vi "Query_Dust_Event.vi"(8 "error in (no error)":errorcluster, 9 "Save Waveforms":bool) -> (0 "error out":errorcluster)   [LabVIEW 2013]
uses:
  Private/Constraints.ctl
  Private/Graph.ctl
  <vilib>/Utility/miscctls.llb/LVPointTypeDef.ctl
  <vilib>/addons/database/Auxilliary.llb/DB Tools Cursor Type.ctl
  <vilib>/Utility/error.llb/DialogType.ctl
  <vilib>/addons/database/Connection.llb/Conn Execute.vi
  <vilib>/addons/database/Recordset.llb/Rec Fetch Recordset Data (R).vi
  <vilib>/addons/database/Recordset.llb/Rec Destroy - Connection.vi
  <userlib>/_OpenG.lib/array/array.llb/Remove Duplicates from 1D Array (String)__ogtk.vi
  <userlib>/_OpenG.lib/array/array.llb/Search 1D Array (String)__ogtk.vi
  <userlib>/_OpenG.lib/array/array.llb/Index 1D Array Elements (String)__ogtk.vi
  <userlib>/_OpenG.lib/array/array.llb/Filter 1D Array (String)__ogtk.vi
  <vilib>/Utility/file.llb/Write To Spreadsheet File (string).vi
  Private/Global graph.vi
  Private/throttle from query.vi
  <userlib>/_OpenG.lib/comparison/comparison.llb/1D String Array Changed__ogtk.vi
  <vilib>/addons/database/_DB Variant To Data/Database Variant To Data.xnode
  <vilib>/addons/database/NI_Database_API.lvlib
panel:
  out "Last Metadata Name":string
  out "Current Limits":T1 {"Dust Quality" scale=0.0..5.0}
  out "Density":dbl
  out "Plotted Cluster":T2 {"Estimate Quality" scale=0.0..5.0; "Lower Mass Limit (kg)" min=-1.0 max=1.0 step=1e-20; "Upper Mass Limit (kg)" min=-1.0 max=1.0 step=1e-20; "Lower Velocity Limit (km/s)" min=-1.0 max=299792000.0; "Upper Velocity Limit (km/s)" min=-1.0 max=299792000.0}
  out "Groups to add":string[](array[string])
  out "Experiments\nto add":string[](array[string])
  out "Reset":bool
  out "Run stop integer timesamp Holder":i64[](array[numeric])
  out "Run start integer timestamp Holder":i64[](array[numeric])
  out "Description Holder":string[](array[string])
  out "Names":string[](array[string])
  in  "write metadata only":bool
  in  "Tab Control":T3(tab)
  in  "Reset Scale to Default":bool
  in  "Reset Limit":bool
  in  "Combine":bool
  out "Plotted Experiment Names":i32(listbox)
  out "Plotted Experiment Groups":i32(listbox)
  in  "Clear Extra Plots":bool
  in  "Experiment Group":string
  in  "Plot":bool
  in  "Search":bool
  in  "Throttle Dust Source After:":i64=9223372036854775807
  in  "Select Names":bool
  in  "Save Metadata":bool
  in  "Show Names":bool
  out "metadata Slide":u8(slide) scale=0.0..100.0
  in  "Save Image":bool
  in  "Plot Radius?":bool
  out "Constrained Distribution":T4
  in  "Experiment Name":string
  out "Slide":u8(slide) scale=0.0..100.0
  in  "Update Plot in Real-time?":bool
  in  "Reset Constraints to Default":bool
  in  "New Plot Window":bool
  out "Number of Matching Events:":i32
  out "Description for Experiment Name:":string caption="Experiment Description:"
  out "Percentage of triggers that fit constraints:":dbl format="%#_4g%"
  out "Total Number of triggers:":i64
  in  "Constraints":T2 {"Estimate Quality" scale=0.0..5.0; "Lower Mass Limit (kg)" min=0.0 step=1e-20; "Upper Mass Limit (kg)" min=0.0 step=1e-20}
  out "Dust Type":string
  in  "Radius (µm)":dbl
  in  "Mass":dbl
  in  "Velocity":dbl
  in  "Update interval (s)":dbl=10.0 min=10.0 max=120.0
  in  "Sensitivity:":dbl=12100000000000.0
  in  "Vnoise Estimate:":dbl=0.005
  in  "Pelletron Voltage (MV):":dbl=2.0
  out "Test":bool caption="Test Database in use:"
  out "Test 2":bool caption="Production Database in use:"
  in  "Exit":bool
  # "Query Dust Event"
  # "Cursor"
  # "Plot Settings:"
  # "Error Status:"
  # "ODBC Connection Status:"
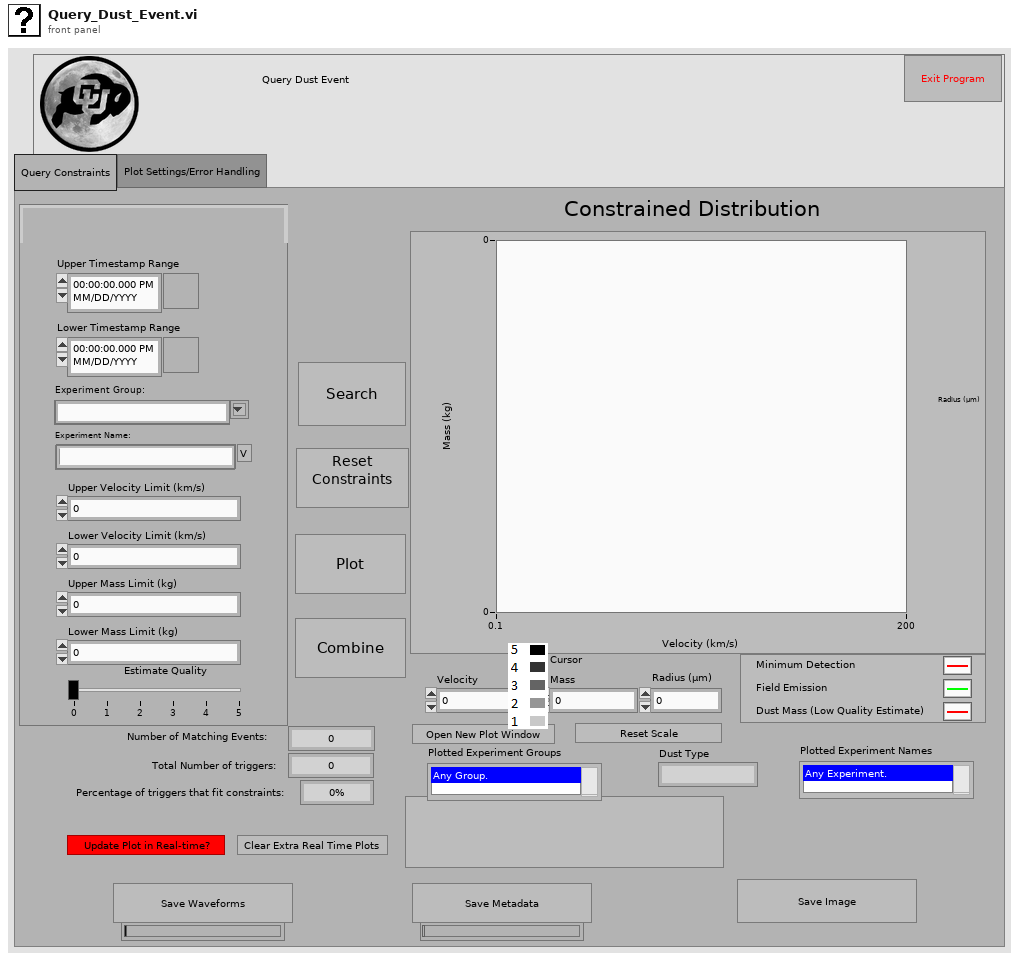
[diagram p1: front panel]
types:
  T1 = cluster{"Lower Timestamp\nRange":timestamp, "Upper Velocity\nLimit (km/s)":dbl, "Lower Velocity\nLimit (km/s)":dbl, "Upper Mass\nLimit (kg)":dbl, "Lower Mass\nLimit (kg)":dbl, "Dust Quality":cluster{i8, i8}}
  T2 = typedef "Constraints.ctl" = cluster{"Upper Timestamp Range":timestamp, "Lower Timestamp Range":timestamp, "Experiment Group:":string, "Experiment Name:":i32[], "Upper Velocity Limit (km/s)":dbl, "Lower Velocity Limit (km/s)":dbl, "Upper Mass Limit (kg)":dbl, "Lower Mass Limit (kg)":dbl, "name array":string[], "Estimate Quality":cluster{dbl, dbl}}
  T3 = enum32{"Query Constraints", "Plot Settings/Error Handling"}
  T4 = typedef "Graph.ctl" = cluster{cluster{"Vnoise":dbl, "Vnoise":dbl}[]}[]
  T5 = typedef "LVPointTypeDef.ctl" = cluster{"Horizontal":i16, "Vertical":i16}
  T6 = enum8{"Enabled", "Disabled", "Disabled and Grayed Out"}
  T7 = typedef "Query_Dust_Event.ctl" = cluster{"Dust Event ID":i64, "Integer Timestamp":i64, "Velocity":sgl, "Mass":sgl, "Charge":sgl, "Radius":sgl, "Passed_3rd_Detector":i8, "High Voltage":sgl, "+ High Voltage Supply":sgl, "- High Voltage Supply":sgl, "HV Control Difference":sgl, "Vacuum Pressure":sgl, "Radiation":sgl, "Column Current":sgl, "Lost Charge":sgl, "Chain Current":sgl, "Control High Voltage":sgl, "Current Group ID:":string, "Current Experiment Name:":string, "Current Experiment Description:":string, "Estimate Source":T8, "Estimate Quality":sgl, "File Location":T9, "Dust Type":string, "Dust Density":sgl}
  T8 = typedef "Estimate_source.ctl" = i8
  T9 = typedef "File_location.ctl" = i8
  T10 = typedef "NI_Database_API.lvlib/DB Tools Cursor Type.ctl" = enum16{"forward-only", "keyset", "dynamic", "static"}
  T11 = enum16{"Left Button", "Center Button", "Right Button", "Window Close"}
  T12 = typedef "NI_Database_API.lvlib/Conn ObjectReference.ctl" = refnum<k1>
  T13 = typedef "NI_Database_API.lvlib/Rec ObjectReference.ctl" = refnum<k1>
  T14 = typedef "DialogType.ctl" = u16
  T15 = typedef "Post_Signal.ctl" = cluster{"Integer Timestamp":i64, "Dust Event ID":i64, "Role ID":T16, "Data":sgl[], "Signal Length":i32, "dt":sgl, "Offset":dbl, "Hardware ID":T17}
  T16 = typedef "Role ID.ctl" = enum16{"First_Detector", "Second_Detector", "Third_Detector", "LeCroy_CH1", "LeCroy_CH2", "LeCroy_CH3", "LeCroy_CH4", "PSU"}
  T17 = typedef "Hardware ID.ctl" = enum16{"Unknown", "CSA 1", "CSA 2", "CSA 3", "CSA 4", "CSA 5", "CSA 6"}
  T18 = typedef "imagedata.ctl" = cluster{"image type":i32, "image depth":i32, "image":u8[], "mask":u8[], "colors":u32[], "Rectangle":cluster{"left":i16, "top":i16, "right":i16, "bottom":i16}}
  T19 = cluster{"Lower Timestamp Range":timestamp, "Upper Velocity Limit (km/s)":dbl, "Lower Velocity Limit (km/s)":dbl, "Upper Mass Limit (kg)":dbl, "Lower Mass Limit (kg)":dbl, "Estimate Quality":cluster{dbl, dbl}}
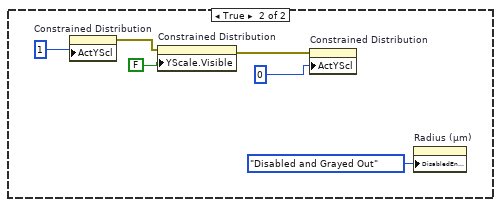
[diagram p2: hidden frame]
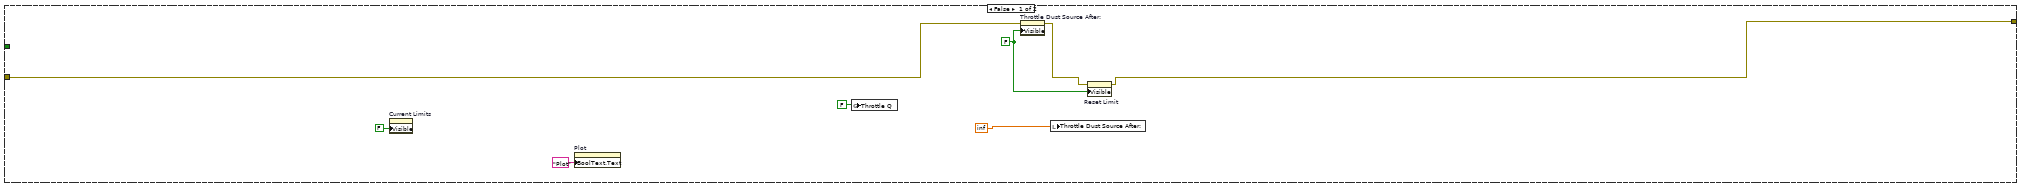
[diagram p5: hidden frame]
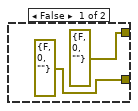
[diagram p6: hidden frame]
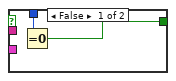
[diagram p7: hidden frame]
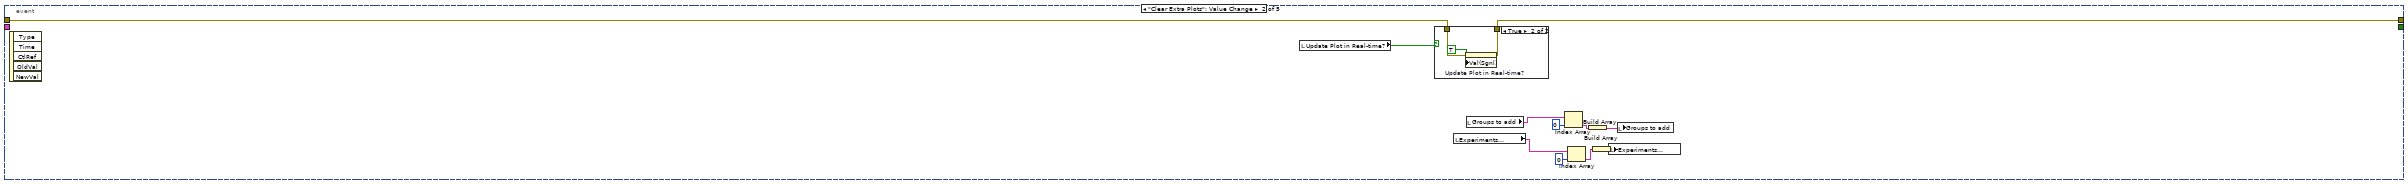
[diagram p8: hidden frame]
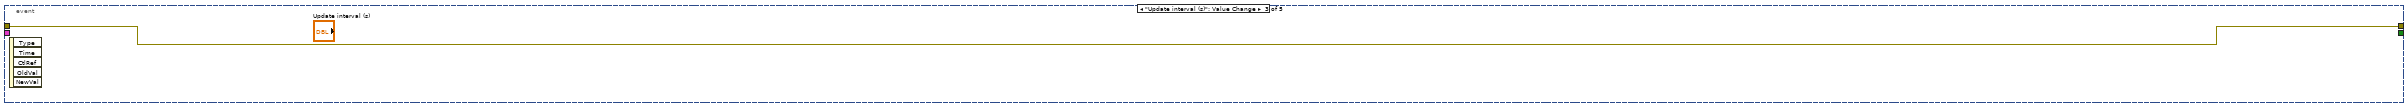
[diagram p10: hidden frame]
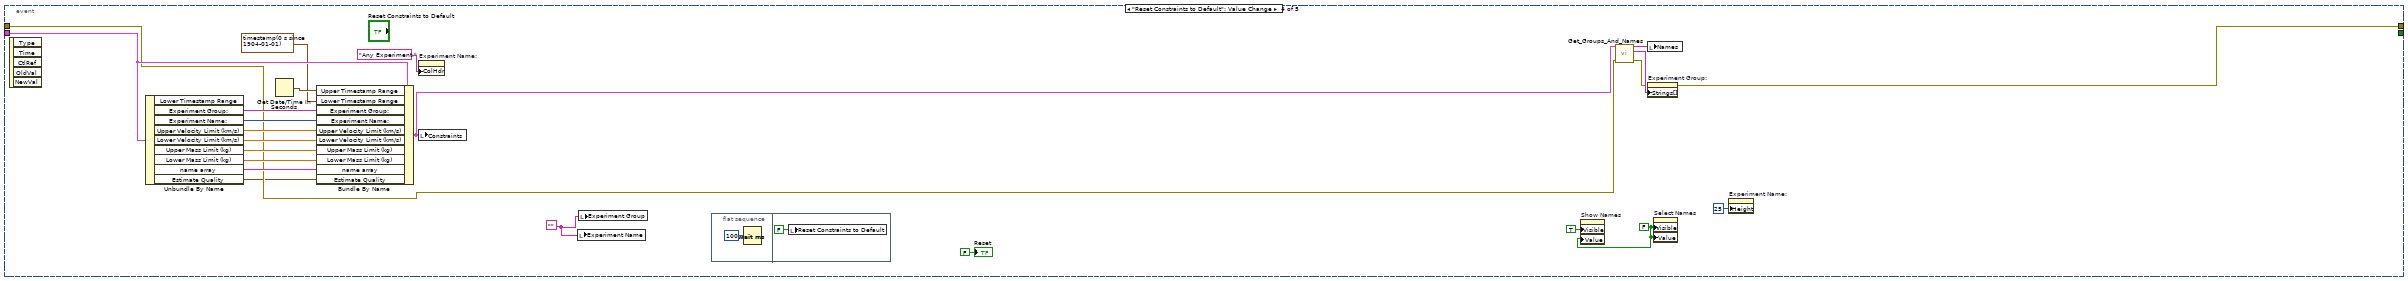
[diagram p11: hidden frame]
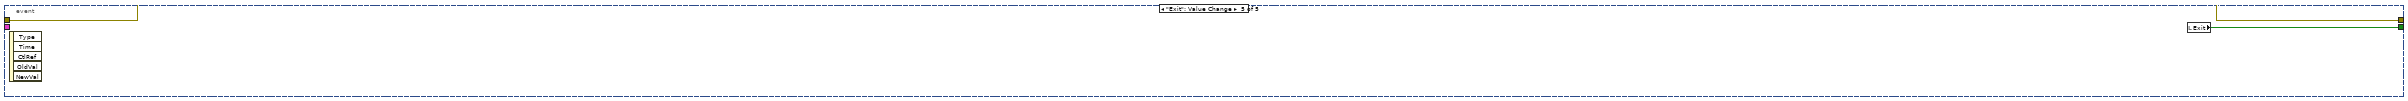
[diagram p12: hidden frame]
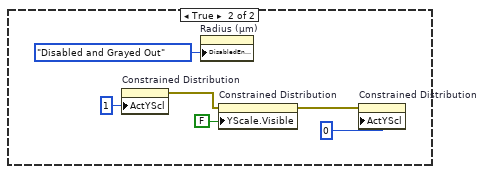
[diagram p15: hidden frame]
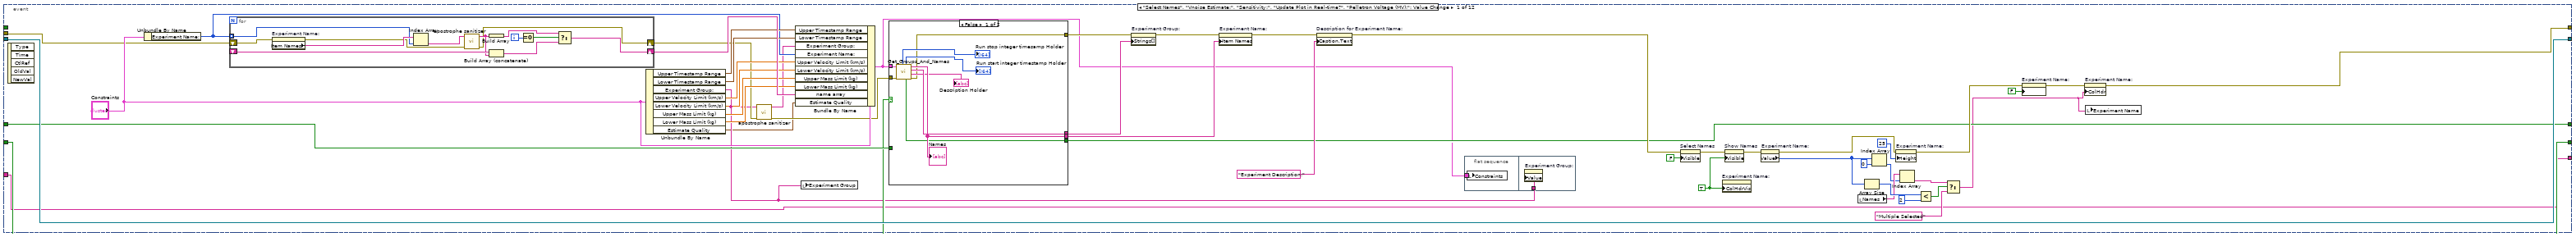
[diagram p16: hidden frame]
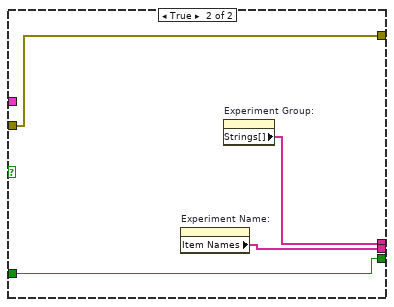
[diagram p17: hidden frame]
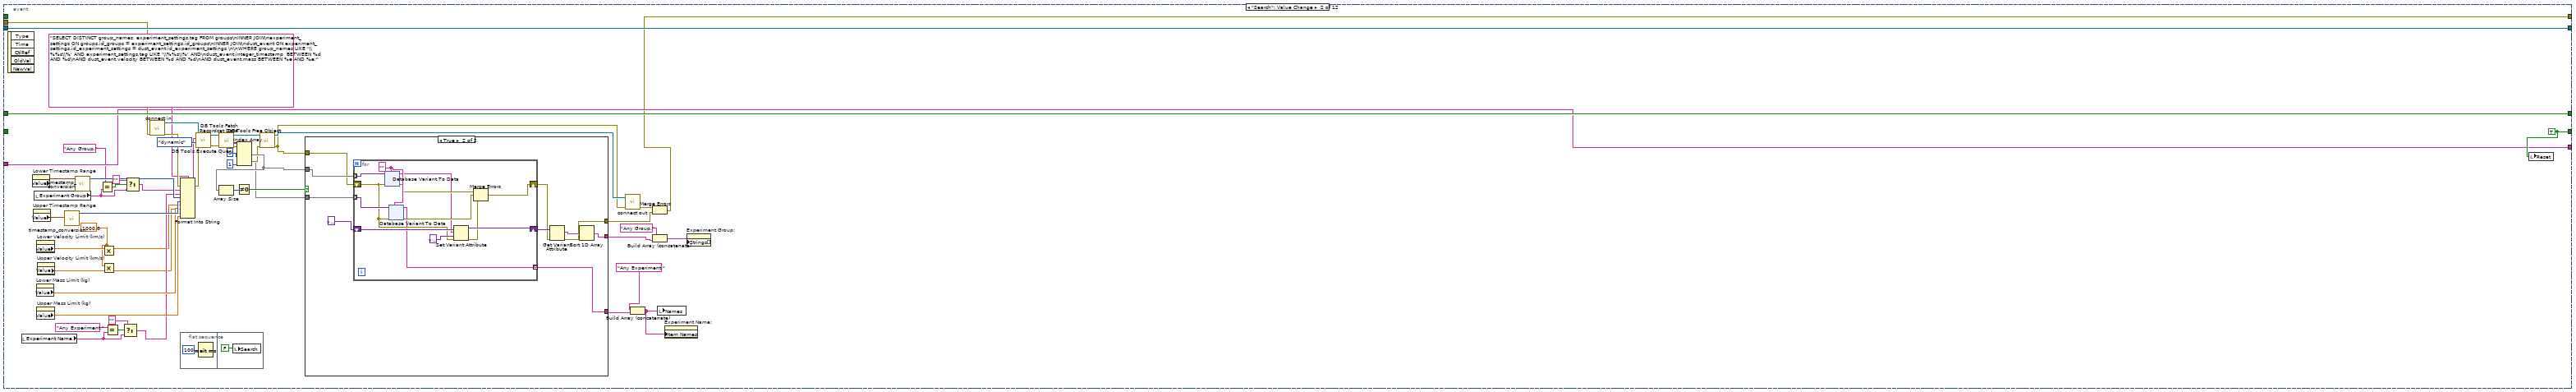
[diagram p18: hidden frame]
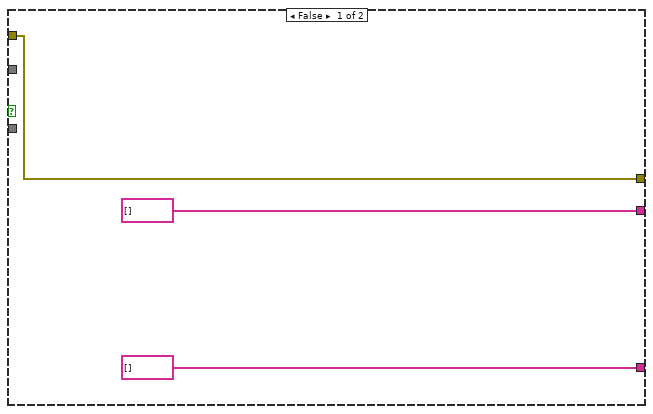
[diagram p19: hidden frame]
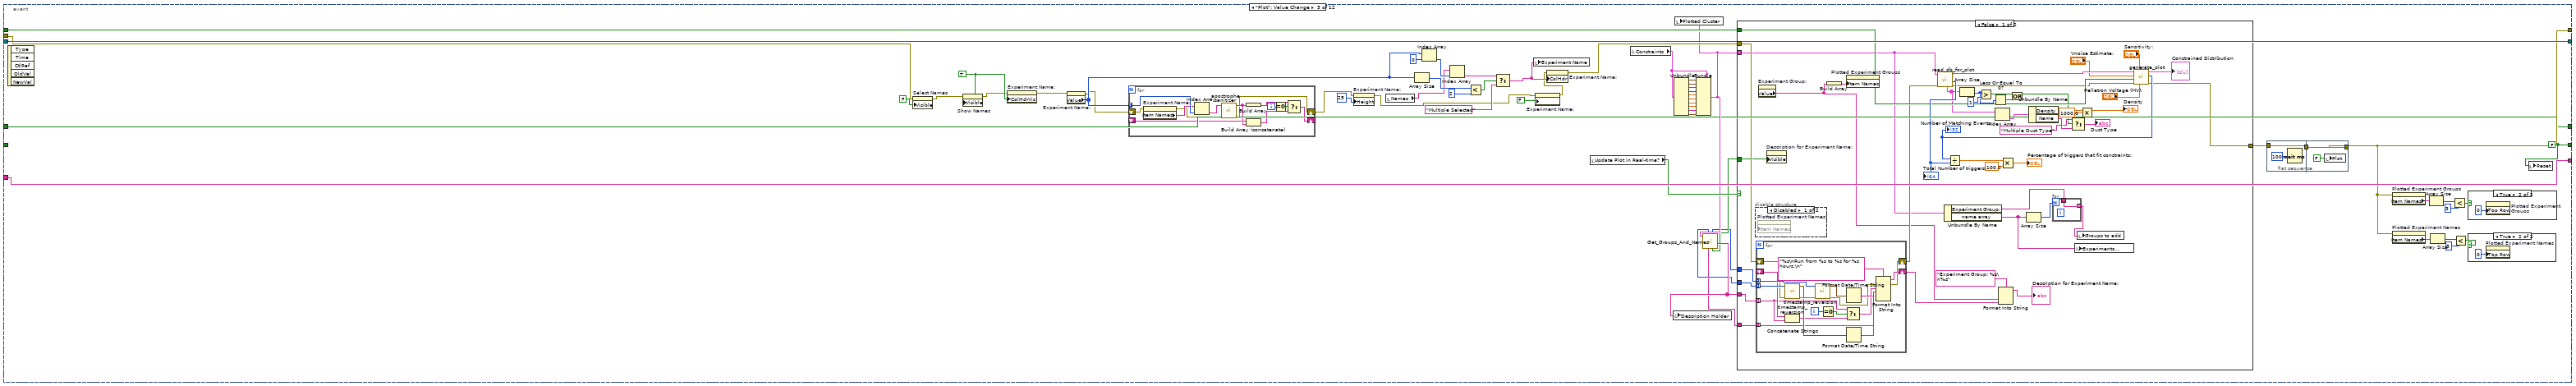
[diagram p20: hidden frame]
diagram:
  w15 = FALSE ("Visible")
  w33 = -1 ("Plotted Experiment Groups")
  w41 = FALSE ("Select Names")
  w24 = string[] ["Any Experiment."] ("Experiment Name:")
  w53 = TRUE ("Visible")
  w57 = FALSE ("Visible")
  w72 = 1
  w77 = 299792
  w64 = FALSE ("write metadata only")
  w83 = 0.005 ("Vnoise")
  w84 = 12100000000000.0 ("Sens")
  w36 = "Any Experiment." ("element")
  w23 = "Any Group." ("element")
  w66 = i64 0 ("Lower Timestamp Limit")
  # "Initialize stuff to everything within the last week"
  n1 = property on="Experiment Group:" class="CmbBox"(error in="error in (no error)", "Value"=w23) -> (error out=w63:errorcluster)  [unwired: 1 in, 1 out]
  n2 = Build Array(w23) -> (w34:string[])
  n3 = Get Date/Time In Seconds() -> (seconds since 1Jan1904=w68:timestamp)
  n4 = property on="Plotted Experiment Groups" class="LstBox (strict)"("Item Names"=w34) -> ()  [unwired: 2 in, 2 out]
  n5 = property on="Upper Timestamp Range" class="AbsTime (strict)"(error in=w63, "Value"=w68) -> (error out=w76:errorcluster)  [unwired: 1 in, 1 out]
  n6 = local write "Experiment Group"(w23) -> ()
  n7 = property on="Upper Velocity Limit (km/s)" class="DigNum (strict)"(error in=w76, "Value"=w77) -> (error out=w75:errorcluster)  [unwired: 1 in, 1 out]
  n8 = local write "metadata Slide"(w66) -> ()
  n9 = property on="Lower Velocity Limit (km/s)" class="DigNum (strict)"(error in=w75, "Value"=w66) -> (error out=w74:errorcluster)  [unwired: 1 in, 1 out]
  n10 = property on="Upper Mass Limit (kg)" class="DigNum (strict)"(error in=w74, "Value"=w72) -> (error out=w73:errorcluster)  [unwired: 1 in, 1 out]
  n11 = property on="Lower Mass Limit (kg)" class="DigNum (strict)"(error in=w73, "Value"=w66) -> (error out=w3:errorcluster)  [unwired: 1 in, 1 out]
  n12 = Subtract(x=timestamp(-2001600 s since 1904-01-01) ("current time"), y=timestamp(-2606400 s since 1904-01-01) ("current time")) -> (x-y=w67:dbl)
  n13 = property on="Experiment Name:" class="LstBox (strict)"(error in=w3, "Height"=25 ("x")) -> (error out=w56:errorcluster)  [unwired: 1 in, 1 out]
  n14 = Build Array(w23) -> (w22:string[])
  n15 = Subtract(x=w68, y=w67) -> (x-y=w65:timestamp)
  n16 = local write "Groups to add"(w22) -> ()
  n17 = property on="Lower Timestamp Range" class="AbsTime (strict)"(error in=w56, "Value"=w65) -> (error out=w60:errorcluster)  [unwired: 1 in, 1 out]
  n18 = local write "Slide"(u8 0 ("Slide")) -> ()
  n19 = property on="Show Names" class="Bool (strict)"("Visible"=TRUE) -> ()  [unwired: 2 in, 2 out]
  n20 = local write "write metadata only"(w64) -> ()
  n21 = local write "New Plot Window"(w64) -> ()
  n22 = local write "Exit"(FALSE) -> ()
  n23 = property on="Show Names" class="Bool (strict)"(error in=w60, "Visible"=w53) -> (error out=w59:errorcluster)  [unwired: 1 in, 1 out]
  n24 = property on="Select Names" class="Bool (strict)"(error in=w59, "Visible"=w57) -> (error out=w58:errorcluster)  [unwired: 1 in, 1 out]
  n25 = local read "Constraints"() -> (w82:T2)
  n26 = property on="Description for Experiment Name:" class="Str"(error in=w58, "Visible"=w57) -> (error out=w5:errorcluster)  [unwired: 1 in, 1 out]
  n27 = Bundle By Name(cluster=w82, "Upper Timestamp Range"=w68, "Lower Timestamp Range"=w65, "Experiment Group:"=w23, "name array"=w24, "Upper Velocity Limit (km/s)"=w77, "Lower Velocity Limit (km/s)"=w66, "Upper Mass Limit (kg)"=w72, "Lower Mass Limit (kg)"=w66, "Experiment Name:"=i32[] [0], "Estimate Quality"=cluster{dbl, dbl} {0.0, 5.0} ("Dust Quality")) -> (w45:T2)
  n28 = local write "Experiments\nto add"(w24) -> ()
  n29 = control-ref of="This VI"() -> (w14:refnum<vi>)
  n30 = property class="VI"(reference=w14) -> (error out=w13:errorcluster, "Panel"=w12:refnum<vi>)  [unwired: 1 in, 1 out]
  n31 = property class="Pnl"(reference=w12, error in=w13) -> (error out=w11:errorcluster, "Panes[]"=w10:refnum<vi>[])  [unwired: 1 out]
  n32 = call "Get_Groups_And_Names.vi"("error in (no error)"=w5, "Constraints"=w45) -> ("error out"=w52:errorcluster, "Groups"=w87:string[], "Names"=w62:string[])  [unwired: 2 in, 5 out]
  n33 = local write "Constraints"(w45) -> ()
  n34 = Build Array(w36) -> (w35:string[])
  n35 = local write "Names"(w62) -> ()
  n36 = local write "Experiment Name"(w36) -> ()
  n37 = Index Array(array=w10, index=0) -> (element=w8:refnum<vi>)
  n38 = property on="Plotted Experiment Names" class="LstBox (strict)"("Item Names"=w35) -> ()  [unwired: 2 in, 2 out]
  n39 = property class="Pane"(reference=w8, error in=w11, "Origin"=T5 {"Horizontal"=0, "Vertical"=0}) -> (error out=w6:errorcluster)  [unwired: 1 out]
  n40 = property on="Experiment Name:" class="LstBox (strict)"(error in=w52, "ColHdrVis"=w53) -> (error out=w51:errorcluster)  [unwired: 1 in, 1 out]
  n41 = property on="Experiment Name:" class="LstBox (strict)"(error in=w51, "ColHdr"=w36) -> (error out=w54:errorcluster)  [unwired: 1 in, 1 out]
  n42 = property on="Experiment Group:" class="CmbBox"(error in=w54, "Strings[]"=w87) -> (error out=w86:errorcluster)  [unwired: 1 in, 1 out]
  n43 = call "read_db_for_plot.vi"("error in (no error)"=w86, "Constraints 2"=w45) -> ("error out"=w85:errorcluster, "Total Number of events"=w47:i64, "Dust Array"=w71:T7[], "Dust Info"=w28:cluster{"Density":dbl, "Name":string}[])  [unwired: 5 in, 1 out]
  n44 = Index Array(array=w28) -> (element=w31:cluster{"Density":dbl, "Name":string})  [unwired: 1 in]
  n45 = Array Size(array=w28) -> (size(s)=w19:i32)
  n46 = Unbundle By Name(w31) -> ("Density"=w25:dbl, "Name"=w30:string)
  n47 = local write "Total Number of triggers:"(w47) -> ()
  n48 = Greater?(x=w19, y=1) -> (0:w26:bool)
  n49 = Less Or Equal To 0?(x=w19) -> (x <= 0?=w20:bool)
  n50 = local write "Sensitivity:"(w84) -> ()
  n51 = local write "Vnoise Estimate:"(w83) -> ()
  n52 = local read "Pelletron Voltage (MV):"() -> (w79:dbl)
  n53 = Multiply(x=1000.0, y=w25) -> (x*y=w2:dbl)
  n54 = Or(x=w26, y=w20) -> (x .or. y?=w21:bool)
  n55 = case shown="False" w21 {
    tunnel: w2 -> [w107 _]
    tunnel: w6 -> [_ _]
    frame False {
      n56 = property on="Constrained Distribution" class="XYGraph (strict)"("ActYScl"=0 ("Active Y Scale")) -> (error out=w104:errorcluster)  [unwired: 2 in, 1 out]
      n57 = property on="Constrained Distribution" class="XYGraph (strict)"(error in=w104) -> (error out=w101:errorcluster, "YScale.Maximum"=w103:dbl, "YScale.Minimum"=w105:dbl)  [unwired: 1 in, 1 out]
      n58 = Multiply(x=w103, y=3.0) -> (x*y=w128:dbl)
      n59 = Multiply(x=w105, y=3.0) -> (x*y=w117:dbl)
      n60 = Divide(x=w128, y=w107) -> (x/y=w127:dbl)
      n61 = Divide(x=w117, y=w107) -> (x/y=w116:dbl)
      n62 = Divide(x=w127, y=4.0) -> (x/y=w125:dbl)
      n63 = Divide(x=w116, y=4.0) -> (x/y=w114:dbl)
      n64 = Reciprocal(x=3.0) -> (1/x=w122:dbl)
      n65 = Reciprocal(x=3.0) -> (1/x=w111:dbl)
      n66 = Divide(x=w125, y=3.141592653589793) -> (x/y=w123:dbl)
      n67 = Divide(x=w114, y=3.141592653589793) -> (x/y=w112:dbl)
      n68 = Power Of X(1:w123, 2:w122) -> (0:w120:dbl)
      n69 = Power Of X(1:w112, 2:w111) -> (0:w109:dbl)
      n70 = property on="Constrained Distribution" class="XYGraph (strict)"(error in=w101, "ActYScl"=1 ("Active Y Scale")) -> (error out=w100:errorcluster)  [unwired: 1 in, 1 out]
      n71 = Multiply(x=w120, y=1000000.0) -> (x*y=w99:dbl)
      n72 = Multiply(x=w109, y=1000000.0) -> (x*y=w98:dbl)
      n73 = property on="Constrained Distribution" class="XYGraph (strict)"(error in=w100, "YScale.Maximum"=w99, "YScale.Minimum"=w98) -> (error out=w96:errorcluster)  [unwired: 1 in, 1 out]
      n74 = property on="Constrained Distribution" class="XYGraph (strict)"(error in=w96, "YScale.Visible"=TRUE ("Y Scale.Visible")) -> (error out=w94:errorcluster)  [unwired: 1 in, 1 out]
      n75 = property on="Constrained Distribution" class="XYGraph (strict)"(error in=w94, "YScale.MarkerVals[]"=dbl[] [0.01, 0.02, 0.05, 0.1, 0.2, 0.5, 1.0, 2.0, 5.0, 10.0] ("Y Scale.Marker Values[]")) -> (error out=w92:errorcluster)  [unwired: 1 in, 1 out]
      n76 = property on="Constrained Distribution" class="XYGraph (strict)"(error in=w92, "ActYScl"=0 ("Active Y Scale")) -> ()  [unwired: 1 in, 2 out]
      n77 = property on="Radius (µm)" class="DigNum (strict)"("DisabledEnum"=T6."Enabled" ("Disabled")) -> ()  [unwired: 2 in, 2 out]
    }
    frame True {
      n78 = property on="Constrained Distribution" class="XYGraph (strict)"("ActYScl"=1 ("Active Y Scale")) -> (error out=w133:errorcluster)  [unwired: 2 in, 1 out]
      n79 = property on="Constrained Distribution" class="XYGraph (strict)"(error in=w133, "YScale.Visible"=FALSE ("Y Scale.Visible")) -> (error out=w131:errorcluster)  [unwired: 1 in, 1 out]
      n80 = property on="Constrained Distribution" class="XYGraph (strict)"(error in=w131, "ActYScl"=0 ("Active Y Scale")) -> ()  [unwired: 1 in, 2 out]
      n81 = property on="Radius (µm)" class="DigNum (strict)"("DisabledEnum"=T6."Disabled and Grayed Out" ("Disabled")) -> ()  [unwired: 2 in, 2 out]
    }
  }
  n82 = Select(t="Multiple Dust Type", s=w21, f=w30) -> (s? t:f=w27:string)
  n83 = local read "Plot Radius?"() -> (w80:bool)
  n84 = local write "Dust Type"(w27) -> ()
  n85 = local write "Density"(w2) -> ()
  n86 = call "generate_plot.vi"("High Voltage"=w79, "Sens"=w84, "error in"=w85, "Plot Radius"=w80, "Vnoise"=w83, "Dust Array"=w71) -> ("error out"=w39:errorcluster, "Number of matching good events"=w46:i32, "Dust Distribution"=w81:T4)  [unwired: 3 in]
  n87 = local write "Number of Matching Events:"(w46) -> ()
  n88 = property on="Upper Timestamp Range" class="AbsTime (strict)"(error in=w39, "DisabledEnum"=T6."Enabled" ("Disabled")) -> (error out=w38:errorcluster)  [unwired: 1 in, 1 out]
  n89 = property on="Plot" class="Bool (strict)"(error in=w38, "BoolText.Text"="Plot" ("Boolean Text.Text")) -> (error out=w18:errorcluster)  [unwired: 1 in, 1 out]
  n90 = local write "Throttle Dust Source After:"(inf) -> ()
  n91 = local write "Select Names"(w41) -> ()
  n92 = local write "Constrained Distribution"(w81) -> ()
  n93 = local write "Update Plot in Real-time?"(w41) -> ()
  n94 = property on="Current Limits" class="Clust (strict)"(error in=w18, "Visible"=w15) -> ()  [unwired: 1 in, 2 out]
  n95 = property on="Plotted Experiment Groups" class="LstBox (strict)"(error in=w18, "Value"=w33) -> ()  [unwired: 1 in, 2 out]
  n96 = property on="Plotted Experiment Names" class="LstBox (strict)"(error in=w18, "Value"=w33) -> ()  [unwired: 1 in, 2 out]
  n97 = property on="Throttle Dust Source After:" class="DigNum (strict)"(error in=w18, "Visible"=w15) -> (error out=w16:errorcluster)  [unwired: 1 in, 1 out]
  n98 = Divide(x=w46, y=w47) -> (x/y=w49:dbl)
  n99 = property on="Experiment Name:" class="LstBox (strict)"(error in=w18, "Top Row"=0) -> (error out=w42:errorcluster)  [unwired: 1 in, 1 out]
  n100 = property on="Reset Limit" class="Bool"(error in=w16, "Visible"=w15) -> ()  [unwired: 1 in, 2 out]
  n101 = case shown="No Error" w42 {
    selector: w42 -> [w141 w1490]
    tunnel: [w148 w1490] -> w89
    tunnel: w45 -> [w146 _]
    frame No Error {
      n102 = call "connect in.vi"("error in (no error)"=w141) -> ("error out"=w149:errorcluster, "Database Connection"=w150:T12, "Test Server"=w138:bool)  [unwired: 6 in]
      "Test" <- w138
      n103 = local read "Experiment Group"() -> (w139:string)
      n104 = property on="Last Metadata Name" class="Str"("Value"="New_Database_Query.csv") -> (error out=w136:errorcluster)  [unwired: 2 in, 1 out]
      n105 = Not(x=w138) -> (.not. x?=→"Test 2":bool)
      n106 = call "connect out.vi"("error in (no error)"=w149, "connection reference"=w150) -> ("error out"=w145:errorcluster)  [unwired: 9 in]
      n107 = while {
        tunnel: w145 -> [w519]
        tunnel: [w513] -> w143
        shift-right: [w509] -> w144
        shift-left: _ -> [w510]
        shift-right: [w508] -> _
        shift-left: _ -> [w507]
        shift-right: [w505] -> _
        shift-left: FALSE -> [w506]
        shift-right: [w503] -> _
        shift-left: w139 -> [w504]
        tunnel: w136 -> [_]
        stop <- "Exit" stop-if-true
        w512 = u8 0 ("Slide")
        w517 = FALSE ("Save to File")
        # "Constraints change/file saving loop"
        n108 = local write "Save Waveforms"(w517) -> ()
        n109 = local write "Save Image"(w517) -> ()
        n110 = local write "Slide"(w512) -> ()
        n111 = local write "Save Metadata"(FALSE ("Save metadata")) -> ()
        n112 = local write "metadata Slide"(w512) -> ()
        n113 = event shown="[3] \"Combine\": Value Change" {
          selector: _ -> [_ _ _ _ _ _ _ _ _ _ _ _]
          dyn-events: _ -> [_ _ _ _ _ _ _ _ _ _ _ _]
          timeout: 100 -> [_ _ _ _ _ _ _ _ _ _ _ _]
          tunnel: w519 -> [w612 w709 w840 w990 w1161 w1180 w1186 _ w1370 w1445 w1460 w1480]
          tunnel: [w598 w675 w814 w991 w1162 w1180 w1200 w1253 w1375 w1445 w1458 w1479] -> w516
          tunnel: "Plot Radius?" -> [_ _ w864 w958 _ _ _ _ _ _ _ _]
          tunnel: w510 -> [w633 w714 w863 w995 w1160 w1179 w1201 w1251 w1374 w1444 w1457 w1476]
          tunnel: [w633 w714 w863 w995 w1160 w1179 w1201 w1251 w1374 w1444 w1457 w1474] -> w509
          tunnel: [w596 w715 w813 w952 w1159 w1178 w1195 w1250 w1373 w1443 w1456 w1473] -> w508
          tunnel: w507 -> [w594 w715 w813 w952 w1159 w1178 w1195 w1250 w1373 w1443 w1456 w1473]
          tunnel: w506 -> [w593 _ _ w994 w1158 w1177 w1194 w1249 w1372 _ w1455 w1472]
          tunnel: [w593 w697 w862 w994 w1158 w1177 w1193 w1249 w1372 w1442 w1455 w1472] -> w505
          tunnel: w504 -> [w592 w679 w859 w993 w1157 w1176 w1191 w1248 w1371 w1441 w1454 w1471]
          tunnel: [w592 w679 w859 w993 w1157 w1176 w1189 w1248 w1371 w1441 w1454 w1471] -> w503
          event "Select Names", "Vnoise Estimate:", "Sensitivity:", "Update Plot in Real-time?", "Pelletron Voltage (MV):": Value Change {
            w607 = TRUE ("Visible")
            n114 = event-data() -> ()  [unwired: 1 in, 5 out]
            n115 = Unbundle By Name("Constraints") -> ("Experiment Name:"=w605:i32[])
            n116 = for {
              tunnel: w605 -> [w660] mode=indexing
              shift-right: [w657] -> w631
              shift-left: _ -> [w659]
              shift-right: [w649] -> w600
              shift-left: w612 -> [w653]
              i -> [w655]
              n117 = property on="Experiment Name:" class="LstBox (strict)"(error in=w653) -> (error out=w650:errorcluster, "Item Names"=w661:string[])  [unwired: 1 in, 1 out]
              n118 = Index Array(array=w661, index=w660) -> (element=w652:string)
              n119 = call "apostrophe sanitizer.vi"("error in (no error)"=w650, "imput to db"=w652) -> ("error out"=w649:errorcluster, "fixed imput to db"=w651:string)  [unwired: 7 in, 1 out]
              n120 = Build Array(w651) -> (w656:string[])
              n121 = Build Array (concatenate)(w659, w651) -> (w658:string[])
              n122 = Equal To 0?(x=w655) -> (x = 0?=w654:bool)
              n123 = Select(t=w656, s=w654, f=w658) -> (s? t:f=w657:string[])
            }
            n124 = Unbundle By Name("Constraints") -> ("Upper Timestamp Range"=w630:timestamp, "Lower Timestamp Range"=w629:timestamp, "Experiment Group:"=w590:string, "Upper Velocity Limit (km/s)"=w628:dbl, "Lower Velocity Limit (km/s)"=w627:dbl, "Upper Mass Limit (kg)"=w626:dbl, "Lower Mass Limit (kg)"=w625:dbl, "Estimate Quality"=w587:cluster{dbl, dbl})
            n125 = call "apostrophe sanitizer.vi"("error in (no error)"=w600, "imput to db"=w590) -> ("error out"=w599:errorcluster, "fixed imput to db"=w601:string)  [unwired: 7 in, 1 out]
            n126 = Bundle By Name(cluster="Constraints", "Upper Timestamp Range"=w630, "Lower Timestamp Range"=w629, "Experiment Group:"=w601, "Experiment Name:"=w605, "Upper Velocity Limit (km/s)"=w628, "Lower Velocity Limit (km/s)"=w627, "Upper Mass Limit (kg)"=w626, "Lower Mass Limit (kg)"=w625, "name array"=w631, "Estimate Quality"=w587) -> (w586:T2)
            n127 = local write "Experiment Group"(w590) -> ()
            n128 = case shown="False" w593 {
              tunnel: [w642 w645] -> w589
              tunnel: [w641 w643] -> w588
              tunnel: w586 -> [w640 _]
              tunnel: w599 -> [w636 w646]
              tunnel: [w635 w644] -> w596
              tunnel: [w634 w646] -> w595
              tunnel: w594 -> [_ w644]
              frame False {
                n129 = call "Get_Groups_And_Names.vi"("error in (no error)"=w636, "Constraints"=w640) -> ("error out"=w634:errorcluster, "Description"=→"Description Holder":string[], "Groups"=w642:string[], "Names"=w641:string[], "Description Returned?"=w635:bool, "Run start integer timestamp"=→"Run start integer timestamp Holder":i64[], "Run stop integer timesamp"=→"Run stop integer timesamp Holder":i64[])  [unwired: 2 in, 1 out]
                "Names" <- w641
              }
              frame True {
                n130 = property on="Experiment Name:" class="LstBox (strict)"() -> ("Item Names"=w643:string[])  [unwired: 2 in, 2 out]
                n131 = property on="Experiment Group:" class="CmbBox"() -> ("Strings[]"=w645:string[])  [unwired: 2 in, 2 out]
              }
            }
            n132 = property on="Experiment Group:" class="CmbBox"(error in=w595, "Strings[]"=w589) -> (error out=w609:errorcluster)  [unwired: 1 in, 1 out]
            n133 = property on="Experiment Name:" class="LstBox (strict)"(error in=w609, "Item Names"=w588) -> (error out=w608:errorcluster)  [unwired: 1 in, 1 out]
            n134 = property on="Description for Experiment Name:" class="Str"(error in=w608, "Caption.Text"="Experiment Description:" ("format string")) -> (error out=w597:errorcluster)  [unwired: 1 in, 1 out]
            n135 = flat-sequence {
              tunnel: w586 -> [w647]
              tunnel: w590 -> [w648]
              frame #0 {
                n136 = local write "Constraints"(w647) -> ()
              }
              frame #1 {
                n137 = property on="Experiment Group:" class="CmbBox"("Value"=w648) -> ()  [unwired: 2 in, 2 out]
              }
            }
            n138 = property on="Select Names" class="Bool (strict)"(error in=w597, "Visible"=FALSE) -> (error out=w613:errorcluster)  [unwired: 1 in, 1 out]
            n139 = property on="Experiment Name:" class="LstBox (strict)"("ColHdrVis"=w607) -> ()  [unwired: 2 in, 2 out]
            n140 = property on="Show Names" class="Bool (strict)"(error in=w613, "Visible"=w607) -> (error out=w611:errorcluster)  [unwired: 1 in, 1 out]
            n141 = property on="Experiment Name:" class="LstBox (strict)"(error in=w611) -> (error out=w610:errorcluster, "Value"=w604:i32[])  [unwired: 1 in, 1 out]
            n142 = local read "Names"() -> (w619:string[])
            n143 = Array Size(array=w604) -> (size(s)=w620:i32)
            n144 = Index Array(array=w604, index=0) -> (element=w606:i32)
            n145 = property on="Experiment Name:" class="LstBox (strict)"(error in=w610, "Height"=u32 25 ("Size:Height")) -> (error out=w615:errorcluster)  [unwired: 1 in, 1 out]
            n146 = Index Array(array=w619, index=w606) -> (element=w602:string)
            n147 = Less?(x=w620, y=2) -> (x < y?=w621:bool)
            n148 = Select(t=w602, s=w621, f="Multiple Selected") -> (s? t:f=w591:string)
            n149 = property on="Experiment Name:" class="LstBox (strict)"(error in=w615, "Scrollbar Visible"=FALSE ("Visible Items:Vertical Scrollbar Visible")) -> (error out=w618:errorcluster)  [unwired: 1 in, 1 out]
            n150 = property on="Experiment Name:" class="LstBox (strict)"(error in=w618, "ColHdr"=w591) -> (error out=w598:errorcluster)  [unwired: 1 in, 1 out]
            n151 = local write "Experiment Name"(w591) -> ()
          }
          event "Search": Value Change {
            w662 = 1000.0 ("y")
            w697 = TRUE
            n152 = event-data() -> ()  [unwired: 1 in, 5 out]
            n153 = local read "Experiment Name"() -> (w666:string)
            n154 = property on="Lower Timestamp Range" class="AbsTime (strict)"() -> ("Value"=w689:timestamp)  [unwired: 2 in, 2 out]
            n155 = property on="Upper Timestamp Range" class="AbsTime (strict)"() -> ("Value"=w690:timestamp)  [unwired: 2 in, 2 out]
            n156 = local read "Experiment Group"() -> (w671:string)
            n157 = property on="Lower Mass Limit (kg)" class="DigNum (strict)"() -> ("Value"=w681:dbl)  [unwired: 2 in, 2 out]
            n158 = property on="Lower Velocity Limit (km/s)" class="DigNum (strict)"() -> ("Value"=w683:dbl)  [unwired: 2 in, 2 out]
            n159 = property on="Upper Mass Limit (kg)" class="DigNum (strict)"() -> ("Value"=w680:dbl)  [unwired: 2 in, 2 out]
            n160 = property on="Upper Velocity Limit (km/s)" class="DigNum (strict)"() -> ("Value"=w682:dbl)  [unwired: 2 in, 2 out]
            n161 = call "timestamp_conversion.vi"("Time Stamp"=w690) -> ("Integer Time"=w684:i64)  [unwired: 8 in, 1 out]
            n162 = call "timestamp_conversion.vi"("Time Stamp"=w689) -> ("Integer Time"=w685:i64)  [unwired: 8 in, 1 out]
            n163 = Equal?(x="Any Group.", y=w671) -> (x = y?=w673:bool)
            n164 = Multiply(x=w683, y=w662) -> (x*y=w664:dbl)
            n165 = Multiply(x=w662, y=w682) -> (x*y=w663:dbl)
            n166 = Equal?(x="Any Experiment.", y=w666) -> (x = y?=w668:bool)
            n167 = Select(t="", s=w668, f=w666) -> (s? t:f=w665:string)
            n168 = Select(t="", s=w673, f=w671) -> (s? t:f=w670:string)
            n169 = call "connect in.vi"("error in (no error)"=w709) -> ("error out"=w708:errorcluster, "Database Connection"=w713:T12)  [unwired: 6 in, 1 out]
            n170 = flat-sequence {
              frame #0 {
                n171 = Wait (ms)(milliseconds to wait=u32 100) -> ()  [unwired: 1 out]
              }
              frame #1 {
                n172 = local write "Search"(FALSE ("Search")) -> ()
              }
            }
            n173 = Format Into String(format string="SELECT DISTINCT group_names, experiment_settings.tag FROM groups\nINNER JOIN\nexperiment_settings ON groups.id_groups = experiment_settings.id_groups\nINNER JOIN\ndust_event ON experiment_settings.id_experiment_settings = dust_event.id_experiment_settings \n\nWHERE group_names LIKE '\\%%s\\%' AND experiment_settings.tag LIKE '\\%%s\\%' AND\ndust_event.integer_timestamp  BETWEEN %d AND %d\nAND dust_event.velocity BETWEEN %d AND %d\nAND dust_event.mass BETWEEN %e AND %e;", error in=w708, w670, w665, w685, w684, w664, w663, w681, w680) -> (resulting string=w706:string, error out=w707:errorcluster)  [unwired: 1 in]
            n174 = call-poly <vilib>:"DB Tools Execute Query.vi"("error in (no error)"=w707, "cursor type"=DB_Tools_Cursor_Type."dynamic", "SQL query"=w706, "connection reference"=w713) -> ("error out"=w711:errorcluster, "recordset reference"=w710:T13)  [unwired: 4 in]
            n175 = call-poly <vilib>:"DB Tools Fetch Recordset Data.vi"("error in (no error)"=w711, "recordset reference"=w710) -> ("error out"=w700:errorcluster, "recordset data"=w705:variant[][], "recordset reference out"=w701:T13)  [unwired: 3 in]
            n176 = Index Array(array=w705, index (col) #1=0 ("index (row)"), index (col) #2=1 ("index (col)")) -> (element #1=w704:variant[], element #2=w686:variant[])  [unwired: 2 in]
            n177 = Array Size(array=w704) -> (size(s)=w702:i32)
            n178 = Not Equal To 0?(x=w702) -> (x != 0?=w703:bool)
            n179 = call-poly <vilib>:"DB Tools Free Object.vi"("error in (no error)"=w700, "recordset reference"=w701) -> ("error out"=w678:errorcluster, "connection reference"=w688:T12)  [unwired: 8 in]
            n180 = case shown="True" w703 {
              tunnel: w704 -> [_ w728]
              tunnel: [string[] [] w722] -> w695
              tunnel: [string[] [] w721] -> w698
              tunnel: w686 -> [_ w727]
              tunnel: w678 -> [w716 w726]
              tunnel: [w716 w719] -> w677
              frame False {
              }
              frame True {
                n181 = for {
                  tunnel: w728 -> [w741] mode=indexing
                  tunnel: w727 -> [w740] mode=indexing
                  shift-right: [w730] -> w720
                  shift-left: w726 -> [w732]
                  shift-right: [w733] -> w724
                  shift-left: variant ("Variant") -> [w736]
                  tunnel: [w729] -> w721 mode=indexing
                  w739 = ""
                  n182 = xnode "Database Variant To Data"("database variant"=w741, "error in (no error)"=w732, "type"=w739) -> ("data"=w735:string, "error out"=w738:errorcluster)
                  n183 = xnode "Database Variant To Data"("database variant"=w740, "error in (no error)"=w732, "type"=w739) -> ("data"=w729:string, "error out"=w737:errorcluster)
                  n184 = Set Variant Attribute(Variant=w736, name=w735, value=variant ("Variant"), error in=w732) -> (Variant out=w733:variant, error out=w731:errorcluster)  [unwired: 1 out]
                  n185 = Merge Errors(w738, w737, w731) -> (w730:errorcluster)
                }
                n186 = Get Variant Attribute(Variant=w724, error in=w720) -> (names=w723:string[], error out=w719:errorcluster)  [unwired: 2 in, 2 out]
                n187 = Sort 1D Array(array=w723) -> (sorted array=w722:string[])
              }
            }
            n188 = call "connect out.vi"("error in (no error)"=w678, "connection reference"=w688) -> ("error out"=w676:errorcluster)  [unwired: 9 in]
            n189 = Build Array (concatenate)("Any Experiment." ("element"), w698) -> (w693:string[])
            n190 = Merge Errors(w676, w677) -> (w675:errorcluster)
            n191 = Build Array (concatenate)("Any Group." ("element"), w695) -> (w696:string[])
            n192 = local write "Names"(w693) -> ()
            n193 = property on="Experiment Name:" class="LstBox (strict)"("Item Names"=w693) -> ()  [unwired: 2 in, 2 out]
            n194 = property on="Experiment Group:" class="CmbBox"("Strings[]"=w696) -> ()  [unwired: 2 in, 2 out]
            n195 = local write "Reset"(w697) -> ()
          }
          event "Plot": Value Change {
            w855 = TRUE ("Visible")
            w862 = FALSE
            n196 = event-data() -> ()  [unwired: 1 in, 5 out]
            n197 = property on="Select Names" class="Bool (strict)"(error in=w840, "Visible"=FALSE) -> (error out=w845:errorcluster)  [unwired: 1 in, 1 out]
            n198 = property on="Show Names" class="Bool (strict)"(error in=w845, "Visible"=w855) -> (error out=w844:errorcluster)  [unwired: 1 in, 1 out]
            n199 = property on="Experiment Name:" class="LstBox (strict)"(error in=w844, "ColHdrVis"=w855) -> (error out=w843:errorcluster)  [unwired: 1 in, 1 out]
            n200 = property on="Experiment Name:" class="LstBox (strict)"(error in=w843) -> (error out=w828:errorcluster, "Value"=w829:i32[])  [unwired: 1 in, 1 out]
            n201 = for {
              tunnel: w829 -> [w879] mode=indexing
              shift-right: [w876] -> _
              shift-left: _ -> [w878]
              shift-right: [w870] -> w827
              shift-left: w828 -> [w867]
              i -> [w874]
              n202 = property on="Experiment Name:" class="LstBox (strict)"(error in=w867) -> (error out=w868:errorcluster, "Item Names"=w869:string[])  [unwired: 1 in, 1 out]
              n203 = Index Array(array=w869, index=w879) -> (element=w872:string)
              n204 = call "apostrophe sanitizer.vi"("error in (no error)"=w868, "imput to db"=w872) -> ("error out"=w870:errorcluster, "fixed imput to db"=w871:string)  [unwired: 7 in, 1 out]
              n205 = Build Array(w871) -> (w875:string[])
              n206 = Build Array (concatenate)(w878, w871) -> (w877:string[])
              n207 = Equal To 0?(x=w874) -> (x = 0?=w873:bool)
              n208 = Select(t=w875, s=w873, f=w877) -> (s? t:f=w876:string[])
            }
            n209 = property on="Experiment Name:" class="LstBox (strict)"(error in=w827, "Height"=u32 25 ("Size:Height")) -> (error out=w842:errorcluster)  [unwired: 1 in, 1 out]
            n210 = local read "Names"() -> (w817:string[])
            n211 = Array Size(array=w829) -> (size(s)=w848:i32)
            n212 = Index Array(array=w829, index=0) -> (element=w850:i32)
            n213 = Index Array(array=w817, index=w850) -> (element=w852:string)
            n214 = Less?(x=w848, y=2) -> (x < y?=w853:bool)
            n215 = Select(t=w852, s=w853, f="Multiple Selected") -> (s? t:f=w857:string)
            n216 = local write "Experiment Name"(w857) -> ()
            n217 = property on="Experiment Name:" class="LstBox (strict)"(error in=w842, "Scrollbar Visible"=FALSE ("Visible Items:Vertical Scrollbar Visible")) -> (error out=w841:errorcluster)  [unwired: 1 in, 1 out]
            n218 = property on="Experiment Name:" class="LstBox (strict)"(error in=w841, "ColHdr"=w857) -> (error out=w839:errorcluster)  [unwired: 1 in, 1 out]
            n219 = local read "Update Plot in Real-time?"() -> (w858:bool)
            n220 = local read "Constraints"() -> (w826:T2)
            n221 = Unbundle(w826) -> ("Upper Timestamp Range"=w838:timestamp, "Lower Timestamp Range"=w837:timestamp, "Experiment Group:"=w836:string, "Experiment Name:"=w835:i32[], "Upper Velocity Limit (km/s)"=w834:dbl, "Lower Velocity Limit (km/s)"=w833:dbl, "Upper Mass Limit (kg)"=w832:dbl, "Lower Mass Limit (kg)"=w831:dbl, "name array"=w830:string[], "Estimate Quality"=w808:cluster{dbl, dbl})
            n222 = Bundle(cluster=w826, "Upper Timestamp Range"=w838, "Lower Timestamp Range"=w837, "Experiment Group:"=w836, "Experiment Name:"=w835, "Upper Velocity Limit (km/s)"=w834, "Lower Velocity Limit (km/s)"=w833, "Upper Mass Limit (kg)"=w832, "Lower Mass Limit (kg)"=w831, "name array"=w830, "Estimate Quality"=w808) -> (w824:T2)
            n223 = local write "Plotted Cluster"(w824) -> ()
            n224 = call "Get_Groups_And_Names.vi"("Constraints"=w824) -> ("Description"=w825:string[], "Description Returned?"=w812:bool, "Run start integer timestamp"=w811:i64[], "Run Time (hrs)"=w809:string[], "Run stop integer timesamp"=w810:i64[])  [unwired: 3 in, 3 out]
            n225 = local write "Description Holder"(w825) -> ()
            n226 = case shown="False" w858 {
              tunnel: w864 -> [w915 _]
              tunnel: w839 -> [w913 w944]
              tunnel: [w911 w944] -> w861
              tunnel: w824 -> [w894 _]
              tunnel: w811 -> [w910 _]
              tunnel: w810 -> [w909 _]
              tunnel: w825 -> [w908 _]
              tunnel: w812 -> [w907 _]
              tunnel: w809 -> [w882 _]
              frame False {
                n227 = disable-structure shown="Disabled" {
                  frame Disabled {
                    n228 = property on="Plotted Experiment Names" class="LstBox (strict)" props=["Item Names"]() -> ()  [unwired: 3 in, 2 out]
                  }
                  frame Enabled {
                  }
                }
                n229 = for {
                  tunnel: w908 -> [w926] mode=indexing
                  tunnel: w909 -> [w941] mode=indexing
                  tunnel: w910 -> [w942] mode=indexing
                  shift-right: [w928] -> w912
                  shift-left: w913 -> [w939]
                  shift-right: [w930] -> w888
                  shift-left: _ -> [w927]
                  tunnel: w882 -> [w924] mode=indexing
                  i -> [w933]
                  n230 = call "timestamp_reversion.vi"("error in (no error)"=w939, "Integer Timestamp"=w941) -> ("error out"=w940:errorcluster, "time stamp"=w937:timestamp)  [unwired: 7 in]
                  n231 = Concatenate Strings(w927, w926) -> (w925:string)
                  n232 = call "timestamp_reversion.vi"("error in (no error)"=w940, "Integer Timestamp"=w942) -> ("error out"=w929:errorcluster, "time stamp"=w938:timestamp)  [unwired: 7 in]
                  n233 = Equal To 0?(x=w933) -> (x = 0?=w931:bool)
                  n234 = Select(t=w926, s=w931, f=w925) -> (s? t:f=w932:string)
                  n235 = Format Date/Time String(seconds (now)=w938) -> (date/time string=w934:string)  [unwired: 2 in]
                  n236 = Format Date/Time String(seconds (now)=w937) -> (date/time string=w935:string)  [unwired: 2 in]
                  n237 = Format Into String(format string="%s\nRun from %s to %s for %s hours.\n", error in=w929, w932, w935, w934, w924) -> (resulting string=w930:string, error out=w928:errorcluster)  [unwired: 1 in]
                }
                n238 = property on="Experiment Group:" class="CmbBox"() -> ("Value"=w887:string)  [unwired: 2 in, 2 out]
                n239 = property on="Description for Experiment Name:" class="Str"("Visible"=w907) -> ()  [unwired: 2 in, 2 out]
                n240 = Build Array(w887) -> (w906:string[])
                n241 = property on="Plotted Experiment Groups" class="LstBox (strict)"("Item Names"=w906) -> ()  [unwired: 2 in, 2 out]
                n242 = call "read_db_for_plot.vi"("error in (no error)"=w912, "Constraints 2"=w894) -> ("error out"=w914:errorcluster, "Total Number of events"=w916:i64, "Dust Array"=w917:T7[], "Dust Info"=w904:cluster{"Density":dbl, "Name":string}[])  [unwired: 5 in, 1 out]
                "Total Number of triggers:" <- w916
                n243 = Unbundle By Name(w894) -> ("Experiment Group:"=w892:string, "name array"=w890:string[])
                n244 = Array Size(array=w904) -> (size(s)=w883:i32)
                n245 = Greater?(x=w883, y=1) -> (0:w898:bool)
                n246 = Less Or Equal To 0?(x=w883) -> (x <= 0?=w884:bool)
                n247 = Index Array(array=w904) -> (element=w903:cluster{"Density":dbl, "Name":string})  [unwired: 1 in]
                n248 = Format Into String(format string="Experiment Group: %s\n%s", w887, w888) -> (resulting string=→"Description for Experiment Name:":string)  [unwired: 2 in, 1 out]
                n249 = Or(x=w898, y=w884) -> (x .or. y?=w885:bool)
                n250 = Array Size(array=w890) -> (size(s)=w893:i32)
                n251 = Unbundle By Name(w903) -> ("Density"=w899:dbl, "Name"=w902:string)
                n252 = for {
                  N: w893 -> [_]
                  tunnel: w892 -> [w923]
                  tunnel: [w923] -> w891 mode=indexing
                }
                n253 = Select(t="Multiple Dust Type", s=w885, f=w902) -> (s? t:f=→"Dust Type":string)
                n254 = local write "Experiments\nto add"(w890) -> ()
                n255 = local write "Groups to add"(w891) -> ()
                n256 = Multiply(x=w899, y=1000.0) -> (x*y=→"Density":dbl)
                n257 = call "generate_plot.vi"("High Voltage"="Pelletron Voltage (MV):", "Sens"="Sensitivity:", "error in"=w914, "Plot Radius"=w915, "Vnoise"="Vnoise Estimate:", "Dust Array"=w917) -> ("error out"=w911:errorcluster, "Number of matching good events"=w918:i32, "Dust Distribution"=→"Constrained Distribution":T4)  [unwired: 3 in]
                "Number of Matching Events:" <- w918
                n258 = Divide(x=w918, y=w916) -> (x/y=w920:dbl)
                n259 = Multiply(x=w920, y=100.0) -> (x*y=→"Percentage of triggers that fit constraints:":dbl)
              }
              frame True {
                n260 = property on="Update Plot in Real-time?" class="Bool (strict)"("Val(Sgnl)"=TRUE ("Value (Signaling)")) -> ()  [unwired: 2 in, 2 out]
              }
            }
            n261 = flat-sequence {
              tunnel: w861 -> [w945]
              tunnel: [w945] -> w860
              tunnel: [w947] -> w814
              tunnel: w860 -> [w947]
              frame #0 {
                n262 = Wait (ms)(milliseconds to wait=u32 100) -> ()  [unwired: 1 out]
              }
              frame #1 {
                n263 = local write "Plot"(FALSE ("Plot")) -> ()
              }
            }
            n264 = property on="Plotted Experiment Groups" class="LstBox (strict)"(error in=w814) -> ("Item Names"=w818:string[])  [unwired: 1 in, 2 out]
            n265 = property on="Plotted Experiment Names" class="LstBox (strict)"(error in=w814) -> ("Item Names"=w819:string[])  [unwired: 1 in, 2 out]
            n266 = Array Size(array=w818) -> (size(s)=w823:i32)
            n267 = Array Size(array=w819) -> (size(s)=w821:i32)
            n268 = Less?(x=w823, y=3) -> (x < y?=w816:bool)
            n269 = Less?(x=w821, y=3) -> (x < y?=w815:bool)
            n270 = case shown="True" w816 {
              frame False {
              }
              frame True {
                n271 = property on="Plotted Experiment Groups" class="LstBox (strict)"("Top Row"=0) -> ()  [unwired: 2 in, 2 out]
              }
            }
            n272 = case shown="True" w815 {
              frame False {
              }
              frame True {
                n273 = property on="Plotted Experiment Names" class="LstBox (strict)"("Top Row"=0) -> ()  [unwired: 2 in, 2 out]
              }
            }
            n274 = local write "Reset"(w862) -> ()
          }
          event "Combine": Value Change {
            w962 = TRUE ("Visible")
            n275 = event-data() -> ()  [unwired: 1 in, 5 out]
            n276 = property on="Select Names" class="Bool (strict)"(error in=w990, "Visible"=FALSE) -> (error out=w961:errorcluster)  [unwired: 1 in, 1 out]
            n277 = property on="Show Names" class="Bool (strict)"(error in=w961, "Visible"=w962) -> (error out=w963:errorcluster)  [unwired: 1 in, 1 out]
            n278 = property on="Experiment Name:" class="LstBox (strict)"(error in=w963, "ColHdrVis"=w962) -> (error out=w964:errorcluster)  [unwired: 1 in, 1 out]
            n279 = property on="Experiment Name:" class="LstBox (strict)"(error in=w964) -> (error out=w965:errorcluster, "Value"=w957:i32[])  [unwired: 1 in, 1 out]
            n280 = for {
              tunnel: w957 -> [w1010] mode=indexing
              shift-right: [w1007] -> _
              shift-left: _ -> [w1009]
              shift-right: [w1001] -> w966
              shift-left: w965 -> [w1000]
              i -> [w1005]
              n281 = property on="Experiment Name:" class="LstBox (strict)"(error in=w1000) -> (error out=w998:errorcluster, "Item Names"=w999:string[])  [unwired: 1 in, 1 out]
              n282 = Index Array(array=w999, index=w1010) -> (element=w1003:string)
              n283 = call "apostrophe sanitizer.vi"("error in (no error)"=w998, "imput to db"=w1003) -> ("error out"=w1001:errorcluster, "fixed imput to db"=w1002:string)  [unwired: 7 in, 1 out]
              n284 = Build Array(w1002) -> (w1006:string[])
              n285 = Build Array (concatenate)(w1009, w1002) -> (w1008:string[])
              n286 = Equal To 0?(x=w1005) -> (x = 0?=w1004:bool)
              n287 = Select(t=w1006, s=w1004, f=w1008) -> (s? t:f=w1007:string[])
            }
            n288 = property on="Experiment Name:" class="LstBox (strict)"(error in=w966, "Height"=u32 25 ("Size:Height")) -> (error out=w977:errorcluster)  [unwired: 1 in, 1 out]
            n289 = local read "Names"() -> (w975:string[])
            n290 = Array Size(array=w957) -> (size(s)=w973:i32)
            n291 = Index Array(array=w957, index=0) -> (element=w971:i32)
            n292 = Index Array(array=w975, index=w971) -> (element=w969:string)
            n293 = Less?(x=w973, y=2) -> (x < y?=w968:bool)
            n294 = Select(t=w969, s=w968, f="Multiple Selected") -> (s? t:f=w978:string)
            n295 = property on="Experiment Name:" class="LstBox (strict)"(error in=w977, "Scrollbar Visible"=FALSE ("Visible Items:Vertical Scrollbar Visible")) -> (error out=w979:errorcluster)  [unwired: 1 in, 1 out]
            n296 = local write "Experiment Name"(w978) -> ()
            n297 = property on="Experiment Name:" class="LstBox (strict)"(error in=w979, "ColHdr"=w978) -> (error out=w960:errorcluster)  [unwired: 1 in, 1 out]
            n298 = local read "Constraints"() -> (w959:T2)
            n299 = local read "Update Plot in Real-time?"() -> (w997:bool)
            n300 = Unbundle(w959) -> ("Upper Timestamp Range"=w980:timestamp, "Lower Timestamp Range"=w981:timestamp, "Experiment Group:"=w982:string, "Experiment Name:"=w983:i32[], "Upper Velocity Limit (km/s)"=w984:dbl, "Lower Velocity Limit (km/s)"=w985:dbl, "Upper Mass Limit (kg)"=w986:dbl, "Lower Mass Limit (kg)"=w987:dbl, "name array"=w988:string[], "Estimate Quality"=w949:cluster{dbl, dbl})
            n301 = Bundle(cluster=w959, "Upper Timestamp Range"=w980, "Lower Timestamp Range"=w981, "Experiment Group:"=w982, "Experiment Name:"=w983, "Upper Velocity Limit (km/s)"=w984, "Lower Velocity Limit (km/s)"=w985, "Upper Mass Limit (kg)"=w986, "Lower Mass Limit (kg)"=w987, "name array"=w988, "Estimate Quality"=w949) -> (w956:T2)
            n302 = call "Get_Groups_And_Names.vi"("Constraints"=w956) -> ("Description"=w996:string[], "Description Returned?"=w951:bool, "Run start integer timestamp"=w954:i64[], "Run Time (hrs)"=w950:string[], "Run stop integer timesamp"=w953:i64[])  [unwired: 3 in, 3 out]
            n303 = local write "Description Holder"(w996) -> ()
            n304 = case shown="False" w997 {
              tunnel: w956 -> [w1046 w1148]
              tunnel: w954 -> [w1078 _]
              tunnel: w953 -> [w1077 _]
              tunnel: w960 -> [w1075 w1136]
              tunnel: w996 -> [w1076 _]
              tunnel: [w1035 w1145] -> w992
              tunnel: w951 -> [w1074 _]
              tunnel: w958 -> [w1073 _]
              tunnel: w950 -> [w1018 _]
              frame False {
                n305 = local read "Groups to add"() -> (w1072:string[])
                n306 = Unbundle By Name(w1046) -> ("Experiment Group:"=w1021:string)
                n307 = local read "Experiments\nto add"() -> (w1053:string[])
                n308 = property on="Plotted Experiment Groups" class="LstBox (strict)"() -> ("Item Names"=w1022:string[])  [unwired: 2 in, 2 out]
                n309 = call-poly <userlib>:"Search Array__ogtk.vi"("Array"=w1072, "Element Data"=w1021) -> ("Indices of Elements"=w1071:i32[])  [unwired: 7 in]
                n310 = Build Array (concatenate)(w1022, w1021) -> (w1020:string[])
                n311 = call-poly <userlib>:"Remove Duplicates from 1D Array__ogtk.vi"("Input Array"=w1020) -> ("Output Array"=w1019:string[])  [unwired: 1 out]
                n312 = call-poly <userlib>:"Index Array Elements__ogtk.vi"("indices"=w1071, "array"=w1053) -> ("elements"=w1057:string[])  [unwired: 9 in]
                n313 = property on="Plotted Experiment Groups" class="LstBox (strict)"("Item Names"=w1019) -> ()  [unwired: 2 in, 2 out]
                n314 = Unbundle By Name(w1046) -> ("name array"=w1058:string[])
                n315 = call-poly <userlib>:"Filter 1D Array__ogtk.vi"("items to filter"=w1057, "array"=w1058) -> ()  [unwired: 4 in, 2 out]
                n316 = property on="Description for Experiment Name:" class="Str"("Visible"=w1074) -> ()  [unwired: 2 in, 2 out]
                n317 = Unbundle(w1046) -> ("Upper Timestamp Range"=w1045:timestamp, "Lower Timestamp Range"=w1044:timestamp, "Experiment Group:"=w1043:string, "Experiment Name:"=w1042:i32[], "Upper Velocity Limit (km/s)"=w1041:dbl, "Lower Velocity Limit (km/s)"=w1040:dbl, "Upper Mass Limit (kg)"=w1039:dbl, "Lower Mass Limit (kg)"=w1038:dbl, "name array"=w1036:string[], "Estimate Quality"=w1015:cluster{dbl, dbl})
                n318 = Bundle(cluster=w1046, "Upper Timestamp Range"=w1045, "Lower Timestamp Range"=w1044, "Experiment Group:"=w1043, "Experiment Name:"=w1042, "Upper Velocity Limit (km/s)"=w1041, "Lower Velocity Limit (km/s)"=w1040, "Upper Mass Limit (kg)"=w1039, "Lower Mass Limit (kg)"=w1038, "name array"=w1036, "Estimate Quality"=w1015) -> (w1037:T2)
                n319 = for {
                  tunnel: w1076 -> [w1116] mode=indexing
                  tunnel: w1077 -> [w1131] mode=indexing
                  tunnel: w1078 -> [w1132] mode=indexing
                  shift-right: [w1118] -> w1026
                  shift-left: w1075 -> [w1129]
                  shift-right: [w1120] -> w1027
                  shift-left: _ -> [w1117]
                  tunnel: w1018 -> [w1114] mode=indexing
                  i -> [w1123]
                  n320 = call "timestamp_reversion.vi"("error in (no error)"=w1129, "Integer Timestamp"=w1131) -> ("error out"=w1130:errorcluster, "time stamp"=w1127:timestamp)  [unwired: 7 in]
                  n321 = Concatenate Strings(w1117, w1116) -> (w1115:string)
                  n322 = call "timestamp_reversion.vi"("error in (no error)"=w1130, "Integer Timestamp"=w1132) -> ("error out"=w1119:errorcluster, "time stamp"=w1128:timestamp)  [unwired: 7 in]
                  n323 = Equal To 0?(x=w1123) -> (x = 0?=w1121:bool)
                  n324 = Select(t=w1116, s=w1121, f=w1115) -> (s? t:f=w1122:string)
                  n325 = Format Date/Time String(seconds (now)=w1128) -> (date/time string=w1124:string)  [unwired: 2 in]
                  n326 = Format Date/Time String(seconds (now)=w1127) -> (date/time string=w1125:string)  [unwired: 2 in]
                  n327 = Format Into String(format string="%s\nRun from %s to %s for %s hours.\n", error in=w1119, w1122, w1125, w1124, w1114) -> (resulting string=w1120:string, error out=w1118:errorcluster)  [unwired: 1 in]
                }
                n328 = call "read_db_for_plot.vi"("error in (no error)"=w1075, "Constraints 2"=w1037) -> ("error out"=w1060:errorcluster, "Total Number of events"=w1051:i64, "Dust Array"=w1061:T7[], "Dust Info"=w1062:cluster{"Density":dbl, "Name":string}[])  [unwired: 5 in, 1 out]
                n329 = Build Array("Any Experiment." ("y")) -> (w1016:string[])
                n330 = local read "Number of Matching Events:"() -> (w1049:i32)
                n331 = local read "Total Number of triggers:"() -> (w1052:i64)
                n332 = Build Array (concatenate)(w1053, w1016) -> (w1032:string[])
                n333 = Array Size(array=w1016) -> (size(s)=w1055:i32)
                n334 = local write "Experiments\nto add"(w1032) -> ()
                n335 = Array Size(array=w1062) -> (size(s)=w1031:i32)
                n336 = local read "Groups to add"() -> (w1056:string[])
                n337 = Greater?(x=w1031, y=1) -> (0:w1067:bool)
                n338 = Equal To 0?(x=w1031) -> (x = 0?=w1030:bool)
                n339 = local read "Description for Experiment Name:"() -> (w1023:string)
                n340 = case shown="False" w1030 {
                  tunnel: w1067 -> [w1110 _]
                  tunnel: w1062 -> [w1104 _]
                  frame False {
                    n341 = Index Array(array=w1104) -> (element=w1107:cluster{"Density":dbl, "Name":string})  [unwired: 1 in]
                    n342 = Unbundle By Name(w1107) -> ("Density"=w1105:dbl, "Name"=w1108:string)
                    n343 = Select(t="Multiple Dust Type", s=w1110, f=w1108) -> (s? t:f=w1106:string)
                    n344 = Multiply(x=1000.0, y=w1105) -> (x*y=w1103:dbl)
                    n345 = local write "Dust Type"(w1106) -> ()
                    n346 = local write "Density"(w1103) -> ()
                  }
                  frame True {
                  }
                }
                n347 = Add(x=w1051, y=w1052) -> (x+y=w1050:i64)
                n348 = local read "Constrained Distribution"() -> (w1034:T4)
                n349 = for {
                  N: w1055 -> [_]
                  shift-right: [w1112] -> w1054
                  shift-left: w1056 -> [w1113]
                  tunnel: w1021 -> [w1111]
                  n350 = Build Array (concatenate)(w1113, w1111) -> (w1112:string[])
                }
                n351 = local write "Total Number of triggers:"(w1050) -> ()
                n352 = Match Pattern(string=w1023, regular expression=w1021) -> (offset past match=w1024:i32)  [unwired: 1 in, 3 out]
                n353 = local write "Groups to add"(w1054) -> ()
                n354 = Less Than 0?(x=w1024) -> (x < 0?=w1017:bool)
                n355 = case shown="True" w1017 {
                  tunnel: w1027 -> [w1080 w1090]
                  tunnel: w1026 -> [_ w1089]
                  tunnel: w1021 -> [_ w1088]
                  tunnel: w1023 -> [_ w1087]
                  tunnel: [w1079 w1086] -> w1025
                  tunnel: w1024 -> [w1083 _]
                  tunnel: w1023 -> [w1081 _]
                  frame False {
                    n356 = Increment(x=w1083) -> (x+1=w1082:i32)
                    n357 = Replace Substring(2:0 ("length (len. of substring)"), 3:w1082, 4:w1080, 5:w1081) -> (1:w1079:string)  [unwired: 1 out]
                  }
                  frame True {
                    n358 = Format Into String(format string="\nExperiment Group: %s\n%s", error in=w1089, w1088, w1090) -> (resulting string=w1085:string)  [unwired: 1 in, 1 out]
                    n359 = Concatenate Strings(w1087, w1085) -> (w1086:string)
                  }
                }
                n360 = local read "Pelletron Voltage (MV):"() -> (w1068:dbl)
                n361 = local write "Description for Experiment Name:"(w1025) -> ()
                n362 = local read "Vnoise Estimate:"() -> (w1070:dbl)
                n363 = local read "Sensitivity:"() -> (w1069:dbl)
                n364 = call "generate_plot.vi"("High Voltage"=w1068, "Sens"=w1069, "error in"=w1060, "Plot Radius"=w1073, "Vnoise"=w1070, "Dust Array"=w1061) -> ("error out"=w1035:errorcluster, "Number of matching good events"=w1048:i32, "Dust Distribution"=w1029:T4)  [unwired: 3 in]
                n365 = Add(x=w1048, y=w1049) -> (x+y=w1047:i32)
                n366 = local write "Number of Matching Events:"(w1047) -> ()
                n367 = Divide(x=w1047, y=w1050) -> (x/y=w1064:dbl)
                n368 = Multiply(x=w1064, y=100.0) -> (x*y=w1065:dbl)
                n369 = Empty Array?(array=w1029) -> (empty?=w1028:bool)
                n370 = case shown="False" w1028 {
                  tunnel: w1034 -> [w1094 w1101]
                  tunnel: w1029 -> [w1093 _]
                  tunnel: [w1092 w1101] -> w1033
                  frame False {
                    n371 = for {
                      tunnel: w1094 -> [w1100] mode=indexing
                      tunnel: w1093 -> [w1099] mode=indexing
                      tunnel: [w1097] -> w1092 mode=indexing
                      n372 = Unbundle(w1100) -> (w1096:cluster{"Vnoise":dbl, "Vnoise":dbl}[])
                      n373 = Unbundle(w1099) -> (w1095:cluster{"Vnoise":dbl, "Vnoise":dbl}[])
                      n374 = Build Array (concatenate)(w1096, w1095) -> (w1098:cluster{"Vnoise":dbl, "Vnoise":dbl}[])
                      n375 = Bundle(w1098) -> (w1097:cluster{cluster{"Vnoise":dbl, "Vnoise":dbl}[]})  [unwired: 1 in]
                    }
                  }
                  frame True {
                  }
                }
                n376 = local write "Percentage of triggers that fit constraints:"(w1065) -> ()
                n377 = local write "Constrained Distribution"(w1033) -> ()
              }
              frame True {
                w1153 = "Any Experiment." ("y")
                n378 = Unbundle By Name(w1148) -> ("Experiment Group:"=w1144:string)
                n379 = Unbundle By Name(w1148) -> ("name array"=w1139:string[])
                n380 = Build Array(w1153) -> (w1150:string[])
                n381 = local read "Experiments\nto add"() -> (w1141:string[])
                n382 = local read "Groups to add"() -> (w1143:string[])
                n383 = call-poly <userlib>:"Search Array__ogtk.vi"("Array"=w1143, "Element Data"=w1144) -> ("Indices of Elements"=w1142:i32[])  [unwired: 7 in]
                n384 = call-poly <userlib>:"Index Array Elements__ogtk.vi"("indices"=w1142, "array"=w1141) -> ("elements"=w1140:string[])  [unwired: 9 in]
                n385 = call-poly <userlib>:"Filter 1D Array__ogtk.vi"("items to filter"=w1140, "array"=w1139) -> ("filtered array"=w1135:string[])  [unwired: 4 in, 1 out]
                n386 = Not Equal?(x=w1135, y=w1153) -> (x != y?=w1147:bool[])
                n387 = Empty Array?(array=w1135) -> (empty?=w1133:bool)
                n388 = Or Array Elements(Boolean array=w1147) -> (logical OR=w1151:bool)
                n389 = Or(x=w1133, y=w1151) -> (x .or. y?=w1134:bool)
                n390 = Select(t=w1135, s=w1134, f=w1150) -> (s? t:f=w1149:string[])
                n391 = Build Array (concatenate)(w1141, w1149) -> (→"Experiments\nto add":string[])
                n392 = Array Size(array=w1149) -> (size(s)=w1138:i32)
                n393 = for {
                  N: w1138 -> [_]
                  shift-right: [w1155] -> w1152
                  shift-left: w1143 -> [w1156]
                  tunnel: w1144 -> [w1154]
                  n394 = Build Array (concatenate)(w1156, w1154) -> (w1155:string[])
                }
                "Groups to add" <- w1152
                n395 = property on="Update Plot in Real-time?" class="Bool (strict)"(error in=w1136, "Val(Sgnl)"=TRUE ("Value (Signaling)")) -> (error out=w1145:errorcluster)  [unwired: 1 in, 1 out]
              }
            }
            n396 = flat-sequence {
              tunnel: w992 -> [w1012]
              tunnel: [w1012] -> w955
              tunnel: [w1013] -> w991
              tunnel: w955 -> [w1013]
              frame #0 {
                n397 = Wait (ms)(milliseconds to wait=u32 100) -> ()  [unwired: 1 out]
              }
              frame #1 {
                n398 = local write "Combine"(FALSE ("Combine")) -> ()
              }
            }
          }
          event "Radius (µm)": Value Change {
            n399 = event-data() -> ()  [unwired: 1 in, 5 out]
            n400 = Divide(x="Radius (µm)", y=1000000.0) -> (x/y=w1167:dbl)
            n401 = local read "Density"() -> (w1164:dbl)
            n402 = Power Of X(1:w1167, 2:3.0 ("y")) -> (0:w1166:dbl)
            n403 = Multiply(x=w1166, y=4.0) -> (x*y=w1174:dbl)
            n404 = Divide(x=w1174, y=3.0) -> (x/y=w1172:dbl)
            n405 = Multiply(x=w1172, y=3.141592653589793) -> (x*y=w1165:dbl)
            n406 = Multiply(x=w1165, y=w1164) -> (x*y=w1163:dbl)
            n407 = property on="Constrained Distribution" class="XYGraph (strict)"(error in=w1161, "Cursor.Cursor Y"=w1163) -> (error out=w1162:errorcluster)  [unwired: 1 in, 1 out]
          }
          event "Mass", "Velocity": Value Change {
            n408 = event-data() -> ()  [unwired: 1 in, 5 out]
            n409 = property on="Constrained Distribution" class="XYGraph (strict)"("Cursor.Cursor X"="Velocity", "Cursor.Cursor Y"="Mass") -> ()  [unwired: 2 in, 2 out]
          }
          event "Show Names": Value Change {
            n410 = event-data() -> ()  [unwired: 1 in, 5 out]
            n411 = property on="Experiment Group:" class="CmbBox"() -> ("Value"=w1189:string)  [unwired: 2 in, 2 out]
            n412 = Equal?(x=w1189, y="Any Group.") -> (x = y?=w1187:bool)
            n413 = Equal?(x=w1189, y=w1191) -> (x = y?=w1192:bool)
            n414 = Or(x=w1192, y=w1187) -> (x .or. y?=w1188:bool)
            n415 = local read "Constraints"() -> (w1196:T2)
            n416 = case shown="True" w1194 {
              selector: w1194 -> [w1220 _]
              tunnel: w1196 -> [w1224 _]
              tunnel: [w1223 w1226] -> w1183
              tunnel: w1186 -> [w1222 w1227]
              tunnel: [w1221 w1227] -> w1185
              tunnel: [w1220 FALSE] -> w1193
              frame False {
                n417 = call "Get_Groups_And_Names.vi"("error in (no error)"=w1222, "Constraints"=w1224) -> ("error out"=w1221:errorcluster, "Names"=w1223:string[])  [unwired: 2 in, 6 out]
              }
              frame True {
                n418 = property on="Experiment Name:" class="LstBox (strict)"() -> ("Item Names"=w1226:string[])  [unwired: 2 in, 2 out]
              }
            }
            n419 = case shown="True" w1188 {
              tunnel: w1185 -> [w1204 w1219]
              tunnel: [w1203 w1216] -> w1184
              tunnel: w1183 -> [_ w1212]
              frame False {
                n420 = property on="Experiment Name:" class="LstBox (strict)"(error in=w1204, "Top Row"=0) -> (error out=w1203:errorcluster)  [unwired: 1 in, 1 out]
              }
              frame True {
                n421 = local read "Experiment Name"() -> (w1218:string)
                n422 = Search 1D Array(1D array=w1212, element=w1218) -> (index of element=w1214:i32)  [unwired: 1 in]
                n423 = Less Than 0?(x=w1214) -> (x < 0?=w1215:bool)
                n424 = Select(t=0, s=w1215, f=w1214) -> (s? t:f=w1208:i32)
                n425 = Subtract(x=w1208, y=5) -> (x-y=w1205:i32)
                n426 = Greater Or Equal To 0?(x=w1205) -> (x >= 0?=w1209:bool)
                n427 = Select(t=w1205, s=w1209, f=0) -> (s? t:f=w1206:i32)
                n428 = property on="Experiment Name:" class="LstBox (strict)"(error in=w1219, "Top Row"=w1206) -> (error out=w1217:errorcluster)  [unwired: 1 in, 1 out]
                n429 = Build Array(w1208) -> (w1211:i32[])
                n430 = property on="Experiment Name:" class="LstBox (strict)"(error in=w1217, "Value"=w1211) -> (error out=w1216:errorcluster)  [unwired: 1 in, 1 out]
              }
            }
            n431 = property on="Experiment Name:" class="LstBox (strict)"("Item Names"=w1183) -> ()  [unwired: 2 in, 2 out]
            n432 = Array Size(array=w1183) -> (size(s)=w1198:i32)
            n433 = Equal?(x=w1198, y=1) -> (x = y?=w1197:bool)
            n434 = case shown="False" w1197 {
              tunnel: w1184 -> [w1235 w1237]
              tunnel: [w1233 w1237] -> w1200
              frame False {
                w1228 = FALSE ("Visible")
                w1232 = TRUE ("Visible Items:Vertical Scrollbar Visible")
                n435 = disable-structure shown="Disabled" {
                  disable-tunnel: w1228 -> [w1236 _]
                  frame Disabled {
                    n436 = property on="Experiment Name:" class="LstBox (strict)"("ColHdrVis"=w1236) -> ()  [unwired: 2 in, 2 out]
                  }
                  frame Enabled {
                  }
                }
                n437 = property on="Show Names" class="Bool (strict)"(error in=w1235, "Visible"=w1228, "Value"=w1228) -> (error out=w1231:errorcluster)  [unwired: 1 in, 1 out]
                n438 = property on="Experiment Name:" class="LstBox (strict)"(error in=w1231, "Scrollbar Visible"=w1232) -> (error out=w1230:errorcluster)  [unwired: 1 in, 1 out]
                n439 = property on="Select Names" class="Bool (strict)"(error in=w1230, "Visible"=w1232) -> (error out=w1234:errorcluster)  [unwired: 1 in, 1 out]
                n440 = property on="Experiment Name:" class="LstBox (strict)"(error in=w1234, "Height"=200 ("x")) -> (error out=w1233:errorcluster)  [unwired: 1 in, 1 out]
              }
              frame True {
              }
            }
          }
          event "Save Waveforms": Value Change {
            w1244 = "*.hdf5"
            n441 = event-data() -> ()  [unwired: 1 in, 5 out]
            n442 = local write "write metadata only"(FALSE) -> ()
            n443 = call "File Dialog"("default name"="New_Database_Query.hdf5", "pattern (all files)"=w1244, "pattern label"=w1244) -> ("selected path"=w1246:path, "exists"=w1240:bool, "cancelled"=w1247:bool, "error out"=w1242:errorcluster)  [unwired: 9 in]
            n444 = Not(x=w1247) -> (.not. x?=w1239:bool)
            n445 = case shown="True" w1240 {
              tunnel: [w1255 w1258] -> w1241
              tunnel: w1242 -> [w1255 w1258]
              tunnel: [TRUE ("T button?") w1257] -> w1238
              frame False {
              }
              frame True {
                n446 = Two Button Dialog(message="Overwrite file?") -> (T button?=w1257:bool)  [unwired: 2 in]
              }
            }
            n447 = And(x=w1239, y=w1238) -> (x .and. y?=w1243:bool)
            n448 = case shown="True" w1243 {
              tunnel: [w1259 w1273] -> w1253
              tunnel: w1241 -> [w1259 w1262]
              tunnel: w1246 -> [_ w1261]
              frame False {
              }
              frame True {
                n449 = local read "Plotted Cluster"() -> (w1260:T2)
                n450 = call "read_db.vi"("error in (no error)"=w1262, "Constraints"=w1260) -> ("error out"=w1274:errorcluster, "Dust Event ID Array"=w1264:i64[], "Dust Array"=w1265:T7[], "File Location Array"=w1263:i64[])  [unwired: 5 in, 1 out]
                n451 = call "open_h5_file.vi"("error in (no error)"=w1274, "path"=w1261) -> ("error out"=w1268:errorcluster, "ref"=w1269:i32)  [unwired: 8 in]
                n452 = disable-structure shown="Enabled" {
                  disable-tunnel: w1269 -> [w1279 w1280]
                  disable-tunnel: w1268 -> [w1278 w1281]
                  disable-tunnel: [w1277 w1281] -> w1267
                  disable-tunnel: [w1276 w1280] -> w1266
                  disable-tunnel: w1265 -> [w1275 _]
                  frame Disabled {
                    n453 = call "Write_summary_file.vi"("Dust Array"=w1275, "error in (no error)"=w1278, "ref"=w1279) -> ("error out"=w1277:errorcluster, "ref out"=w1276:i32)  [unwired: 7 in]
                  }
                  frame Enabled {
                  }
                }
                n454 = for {
                  tunnel: w1264 -> [w1284] mode=indexing
                  shift-right: [w1288] -> w1271
                  shift-left: w1267 -> [w1285]
                  shift-right: [w1286] -> w1270
                  shift-left: w1266 -> [w1287]
                  tunnel: w1263 -> [w1282] mode=indexing
                  i -> [w1283]
                  n455 = case shown="No Error" w1285 {
                    selector: w1285 -> [w1300 w1358]
                    tunnel: [w1291 w1358] -> w1288
                    tunnel: w1287 -> [w1311 w1357]
                    tunnel: [w1309 w1357] -> w1286
                    tunnel: w1284 -> [w1298 _]
                    tunnel: w1283 -> [w1305 _]
                    tunnel: w1282 -> [w1289 _]
                    frame No Error {
                      w1299 = T14 0 items=["no dialog", "OK message", "continue or stop message", "OK message + warnings", "continue/stop + warnings"] ("type of dialog (OK msg:1)")
                      n456 = call "read_signal.vi"("error in (no error)"=w1300, "Location"=w1289, "Dust Event ID"=w1298) -> ("error out"=w1302:errorcluster, "Signal Array"=w1310:T15[])  [unwired: 7 in]
                      n457 = call <vilib>:"General Error Handler.vi"("type of dialog (OK msg:1)"=w1299, "error in (no error)"=w1302) -> ("error?"=w1297:bool, "error out"=w1301:errorcluster)  [unwired: 9 in, 3 out]
                      n458 = case shown="True" w1297 {
                        tunnel: [w1317 w1319] -> w1292
                        tunnel: w1311 -> [w1316 w1322]
                        tunnel: w1310 -> [w1315 _]
                        tunnel: [w1314 w1321] -> w1309
                        tunnel: w1305 -> [w1313 w1323]
                        tunnel: w1301 -> [w1312 w1325]
                        tunnel: w1298 -> [_ w1320]
                        frame False {
                          n459 = call "Write_signals_file.vi"("Index"=w1313, "Signal Array"=w1315, "error in (no error)"=w1312, "ref"=w1316) -> ("error out"=w1317:errorcluster, "ref out"=w1314:i32)  [unwired: 6 in]
                        }
                        frame True {
                          n460 = local read "write metadata only"() -> (w1318:bool)
                          n461 = case shown="False" w1318 {
                            tunnel: [w1331 T11."Center Button" ("Which Button?")] -> w1324
                            frame False {
                              n462 = call <vilib>:"Three Button Dialog.vi"("Allow user to close window? (TRUE)"=FALSE, "Right Button Text (\"Cancel\")"="Cancel" ("F button name (\"Cancel\")"), "Center Button Text (\"No\")"="Continue for all events in dataset" ("F button name (\"Cancel\")"), "Left Button Text (\"Yes\")"="Continue for this event" ("T button name (\"OK\")"), "message"="Waveform not found!") -> ("Which Button?"=w1331:T11)  [unwired: 6 in]
                            }
                            frame True {
                            }
                          }
                          n463 = case shown="\"Center Button\"" w1324 {
                            tunnel: w1325 -> [w1340 w1350 w1354]
                            tunnel: [w1337 w1347 w1353] -> w1319
                            tunnel: w1322 -> [w1338 w1348 w1352]
                            tunnel: w1323 -> [w1341 w1351 _]
                            tunnel: [w1339 w1349 w1352] -> w1321
                            tunnel: w1320 -> [w1334 w1344 _]
                            frame "Left Button", Default {
                              n464 = call <vilib>:"Clear Errors.vi"("error in (no error)"=w1340) -> ("error out"=w1335:errorcluster)  [unwired: 6 in]
                              n465 = call "get_timestamp.vi"("error in (no error)"=w1335, "Index"=w1334) -> ("error out"=w1336:errorcluster, "Signal Array"=w1333:T15[])  [unwired: 8 in]
                              n466 = call "Write_signals_file.vi"("Index"=w1341, "Signal Array"=w1333, "error in (no error)"=w1336, "ref"=w1338) -> ("error out"=w1337:errorcluster, "ref out"=w1339:i32)  [unwired: 6 in]
                            }
                            frame "Center Button" {
                              n467 = call <vilib>:"Clear Errors.vi"("error in (no error)"=w1350) -> ("error out"=w1345:errorcluster)  [unwired: 6 in]
                              n468 = local write "write metadata only"(TRUE) -> ()
                              n469 = call "get_timestamp.vi"("error in (no error)"=w1345, "Index"=w1344) -> ("error out"=w1346:errorcluster, "Signal Array"=w1343:T15[])  [unwired: 8 in]
                              n470 = call "Write_signals_file.vi"("Index"=w1351, "Signal Array"=w1343, "error in (no error)"=w1346, "ref"=w1348) -> ("error out"=w1347:errorcluster, "ref out"=w1349:i32)  [unwired: 6 in]
                            }
                            frame "Right Button" {
                              n471 = call <vilib>:"Clear Errors.vi"("error in (no error)"=w1354) -> ("error out"=w1356:errorcluster)  [unwired: 6 in]
                              n472 = call "Close_H5_file.vi"("error in (no error)"=w1356, "ref"=w1352) -> ("error out"=w1355:errorcluster)  [unwired: 9 in]
                              n473 = Merge Errors(w1355, w1354) -> (w1353:errorcluster)
                            }
                          }
                        }
                      }
                      n474 = local read "Number of Matching Events:"() -> (w1308:i32)
                      n475 = Add(x=1, y=w1305) -> (x+y=w1304:i32)
                      n476 = Divide(x=w1304, y=w1308) -> (x/y=w1307:dbl)
                      n477 = Multiply(x=w1307, y=100) -> (x*y=w1293:dbl)
                      "Slide" <- w1293
                      n478 = Number To Decimal String(number=w1293) -> (decimal integer string=w1296:string)  [unwired: 1 in]
                      n479 = Concatenate Strings("Writing...\n" ("string"), w1296, "% Complete." ("string")) -> (w1290:string)
                      n480 = property on="Save Waveforms" class="Bool (strict)"(error in=w1292, "BoolText.Text"=w1290) -> (error out=w1291:errorcluster)  [unwired: 1 in, 1 out]
                    }
                    frame Error {
                    }
                  }
                }
                n481 = call "Close_H5_file.vi"("error in (no error)"=w1267, "ref"=w1270) -> ("error out"=w1272:errorcluster)  [unwired: 9 in]
                n482 = Merge Errors(w1271, w1272) -> (w1273:errorcluster)
                n483 = local write "error out"(w1273) -> ()
              }
            }
          }
          event "Save Metadata": Value Change {
            w1368 = "*.csv"
            n484 = event-data() -> ()  [unwired: 1 in, 5 out]
            n485 = local read "Last Metadata Name"() -> (w1365:string)
            n486 = call "File Dialog"("default name"=w1365, "error in"=w1370, "pattern (all files)"=w1368, "pattern label"=w1368) -> ("selected path"=w1367:path, "exists"=w1364:bool, "cancelled"=w1369:bool, "error out"=w1363:errorcluster)  [unwired: 8 in]
            n487 = case shown="True" w1364 {
              tunnel: [w1377 w1380] -> w1362
              tunnel: w1363 -> [w1377 w1380]
              tunnel: [TRUE ("T button?") w1379] -> w1359
              frame False {
              }
              frame True {
                n488 = Two Button Dialog(message="Overwrite file?") -> (T button?=w1379:bool)  [unwired: 2 in]
              }
            }
            n489 = Strip Path(path=w1367) -> (name=→"Last Metadata Name":string)  [unwired: 1 out]
            n490 = Not(x=w1369) -> (.not. x?=w1361:bool)
            n491 = And(x=w1361, y=w1359) -> (x .and. y?=w1360:bool)
            n492 = case shown="True" w1360 {
              tunnel: w1367 -> [_ w1394]
              tunnel: w1362 -> [w1381 w1384]
              tunnel: [w1381 w1390] -> w1375
              frame False {
              }
              frame True {
                n493 = local read "Plotted Cluster"() -> (w1385:T2)
                n494 = property on="Save Metadata" class="Bool (strict)"(error in=w1384, "BoolText.Text"="Querying Database\n(may take several mins)" ("Boolean Text.Text")) -> (error out=w1383:errorcluster)  [unwired: 1 in, 1 out]
                n495 = call "read_db.vi"("error in (no error)"=w1383, "Constraints"=w1385) -> ("error out"=w1391:errorcluster, "Dust Array"=w1393:T7[])  [unwired: 5 in, 3 out]
                n496 = Array Size(array=w1393) -> (size(s)=w1392:i32)
                n497 = for {
                  tunnel: w1393 -> [w1440] mode=indexing
                  tunnel: w1392 -> [w1423]
                  shift-right: [w1422] -> w1390
                  shift-left: w1391 -> [w1413]
                  tunnel: [w1409] -> w1387 mode=indexing
                  i -> [w1424]
                  w1400 = "\" %s \"" ("format string")
                  w1398 = "%Y%m%d%H%M%S%9u" ("time format string (%c)")
                  n498 = Add(x=1, y=w1424) -> (x+y=w1427:i32)
                  n499 = Divide(x=w1427, y=w1423) -> (x/y=w1425:dbl)
                  n500 = Unbundle By Name(w1440) -> ("Dust Event ID"=w1421:i64, "Integer Timestamp"=w1414:i64, "Velocity"=w1420:sgl, "Mass"=w1419:sgl, "Charge"=w1415:sgl, "Radius"=w1418:sgl, "High Voltage"=w1417:sgl, "Current Group ID:"=w1404:string, "Current Experiment Name:"=w1406:string, "Current Experiment Description:"=w1408:string, "Estimate Quality"=w1416:sgl, "Dust Type"=w1402:string)
                  n501 = Multiply(x=w1425, y=100) -> (x*y=w1411:dbl)
                  "metadata Slide" <- w1411
                  n502 = call "timestamp_reversion.vi"("error in (no error)"=w1413, "Integer Timestamp"=w1414) -> ("error out"=w1412:errorcluster, "time stamp"=w1397:timestamp)  [unwired: 7 in]
                  n503 = Number To Decimal String(number=w1411) -> (decimal integer string=w1429:string)  [unwired: 1 in]
                  n504 = Concatenate Strings("Writing...\n" ("string"), w1429, "% Complete." ("string")) -> (w1432:string)
                  n505 = Format Date/Time String(time format string (%c)=w1398, seconds (now)=w1397) -> (date/time string=w1410:string)  [unwired: 1 in]
                  n506 = Format Into String(format string=w1400, w1404) -> (resulting string=w1403:string)  [unwired: 2 in, 1 out]
                  n507 = Format Into String(format string=w1400, w1406) -> (resulting string=w1405:string)  [unwired: 2 in, 1 out]
                  n508 = Format Into String(format string=w1400, w1408) -> (resulting string=w1407:string)  [unwired: 2 in, 1 out]
                  n509 = Format Into String(format string=w1400, w1402) -> (resulting string=w1401:string)  [unwired: 2 in, 1 out]
                  n510 = Number To Decimal String(number=w1421) -> (decimal integer string=w1399:string)  [unwired: 1 in]
                  n511 = Number To Decimal String(number=w1414) -> (decimal integer string=w1439:string)  [unwired: 1 in]
                  n512 = Number To Exponential String(number=w1420) -> (E-format string=w1438:string)  [unwired: 3 in]
                  n513 = Number To Exponential String(number=w1419) -> (E-format string=w1437:string)  [unwired: 3 in]
                  n514 = Number To Exponential String(number=w1415) -> (E-format string=w1436:string)  [unwired: 3 in]
                  n515 = Number To Exponential String(number=w1418) -> (E-format string=w1435:string)  [unwired: 3 in]
                  n516 = Number To Exponential String(number=w1417) -> (E-format string=w1434:string)  [unwired: 3 in]
                  n517 = Number To Decimal String(number=w1416) -> (decimal integer string=w1433:string)  [unwired: 1 in]
                  n518 = Format Date/Time String(time format string (%c)=w1398, seconds (now)=w1397, UTC format=TRUE) -> (date/time string=w1395:string)
                  n519 = property on="Save Metadata" class="Bool (strict)"(error in=w1412, "BoolText.Text"=w1432) -> (error out=w1422:errorcluster)  [unwired: 1 in, 1 out]
                  n520 = Build Array(w1399, w1395, w1410, w1439, w1438, w1437, w1436, w1435, w1434, w1403, w1405, w1407, w1433, w1401) -> (w1409:string[])
                }
                n521 = Build Array (concatenate)(string[] ["Dust Event ID", "UTC Timestamp", "Local Timestamp", "Integer Timestamp (ms)", "Velocity (m/s)", "Mass (kg)", "Charge (C)", "Radius (m) ", "High Voltage (MV)", "Current Group ID", "Current Experiment Name", "Current Experiment Description", "Estimate Quality", "Dust Type", "Dust Type", "Dust Type"], w1387) -> (w1386:string[][])
                n522 = call-poly <vilib>:"Write To Spreadsheet File.vi"("delimiter (\\t)"="," ("delimiter (\\t)"), "2D data"=w1386, "file path (dialog if empty)"=w1394) -> ()  [unwired: 5 in, 1 out]
              }
            }
          }
          event Timeout {
            n523 = event-data() -> ()  [unwired: 1 in, 2 out]
            n524 = local read "Reset"() -> (w1442:bool)
          }
          event "Save Image": Value Change {
            w1450 = "*.png"
            n525 = event-data() -> ()  [unwired: 1 in, 5 out]
            n526 = invoke on="Constrained Distribution" class="XYGraph (strict)" method="Get Image"(error in=w1460) -> (error out=w1451:errorcluster, "image data"=w1459:T18)  [unwired: 5 in, 4 out]
            n527 = call "File Dialog"("default name"="Distribution.png", "error in"=w1451, "pattern (all files)"=w1450, "pattern label"=w1450) -> ("selected path"=w1453:path, "exists"=w1447:bool, "error out"=w1448:errorcluster)  [unwired: 8 in, 1 out]
            n528 = case shown="True" w1447 {
              tunnel: [w1467 w1470] -> w1449
              tunnel: w1448 -> [w1467 w1470]
              tunnel: [TRUE ("T button?") w1469] -> w1446
              frame False {
              }
              frame True {
                n529 = Two Button Dialog(message="Overwrite file?") -> (T button?=w1469:bool)  [unwired: 2 in]
              }
            }
            n530 = case shown="False" w1446 {
              tunnel: w1459 -> [_ w1465]
              tunnel: [w1461 w1464] -> w1458
              tunnel: w1453 -> [_ w1463]
              tunnel: w1449 -> [w1461 w1462]
              frame False {
              }
              frame True {
                n531 = call <vilib>:"Write PNG File.vi"("error in (no error)"=w1462, "image data"=w1465, "path to PNG file"=w1463) -> ("error out"=w1464:errorcluster)  [unwired: 7 in, 1 out]
              }
            }
          }
          event "New Plot Window": Value Change {
            w1478 = FALSE ("Wait Until Done")
            n532 = event-data() -> ()  [unwired: 1 in, 5 out]
            n533 = local read "Constrained Distribution"() -> (w1477:T4)
            n534 = global write "Global graph.vi" "Dust Distribution"(w1477) -> ()
            n535 = call "constants.vi"("error in (no error)"=w1480) -> ("error out"=w1488:errorcluster, "Private Folder file path"=w1485:path)  [unwired: 4 in, 5 out]
            n536 = Build Path(base path=w1485, name or relative path="show_new_plot.vit") -> (appended path=w1486:path)
            n537 = Open VI Reference(vi path=w1486, error in (no error)=w1488) -> (vi reference=w1484:refnum<vi>, error out=w1489:errorcluster)  [unwired: 4 in]
            n538 = property class="VI"(reference=w1484, error in=w1489, "Front Panel.Open"=TRUE ("Front Panel Window:Open")) -> (reference out=w1481:refnum<vi>, error out=w1482:errorcluster)
            n539 = local write "New Plot Window"(w1478) -> ()
            n540 = invoke class="VI" method="Run VI"(reference=w1481, error in=w1482, "Wait until done"=w1478, "Auto Dispose Ref"=w1478) -> (reference out=w1475:refnum<vi>, error out=w1479:errorcluster)  [unwired: 1 in, 3 out]
            n541 = Build Array (concatenate)(w1475, w1476) -> (w1474:refnum<vi>[])
          }
        }
        n542 = property on="Constrained Distribution" class="XYGraph (strict)"() -> ("Cursor.Cursor Y"=w498:dbl, "Cursor.Cursor X"=w499:dbl)  [unwired: 2 in, 2 out]
        n543 = local read "Dust Type"() -> (w502:string)
        n544 = local write "Velocity"(w499) -> ()
        n545 = local write "Mass"(w498) -> ()
        n546 = Equal?(x=w502, y="Multiple Dust Type" ("t")) -> (x = y?=w500:bool)
        n547 = case shown="False" w500 {
          tunnel: w498 -> [w528 _]
          frame False {
            n548 = local read "Density"() -> (w527:dbl)
            n549 = Multiply(x=w528, y=3.0) -> (x*y=w578:dbl)
            n550 = Divide(x=w578, y=w527) -> (x/y=w577:dbl)
            n551 = Divide(x=w577, y=4.0) -> (x/y=w576:dbl)
            n552 = Reciprocal(x=3.0) -> (1/x=w573:dbl)
            n553 = Divide(x=w576, y=3.141592653589793) -> (x/y=w574:dbl)
            n554 = Power Of X(1:w574, 2:w573) -> (0:w571:dbl)
            n555 = Multiply(x=w571, y=1000000.0) -> (x*y=w568:dbl)
            n556 = local write "Radius (µm)"(w568) -> ()
            n557 = property on="Radius (µm)" class="DigNum (strict)"("DisabledEnum"=T6."Enabled" ("Disabled")) -> ()  [unwired: 2 in, 2 out]
            n558 = property on="Constrained Distribution" class="XYGraph (strict)"("ActYScl"=0 ("Active Y Scale")) -> (error out=w532:errorcluster)  [unwired: 2 in, 1 out]
            n559 = property on="Constrained Distribution" class="XYGraph (strict)"(error in=w532) -> (error out=w557:errorcluster, "YScale.Maximum"=w555:dbl, "YScale.Minimum"=w556:dbl)  [unwired: 1 in, 1 out]
            n560 = Multiply(x=w555, y=3.0) -> (x*y=w534:dbl)
            n561 = Multiply(x=w556, y=3.0) -> (x*y=w545:dbl)
            n562 = Divide(x=w534, y=w527) -> (x/y=w535:dbl)
            n563 = Divide(x=w545, y=w527) -> (x/y=w546:dbl)
            n564 = Divide(x=w535, y=4.0) -> (x/y=w537:dbl)
            n565 = Divide(x=w546, y=4.0) -> (x/y=w548:dbl)
            n566 = Reciprocal(x=3.0) -> (1/x=w540:dbl)
            n567 = Reciprocal(x=3.0) -> (1/x=w551:dbl)
            n568 = Divide(x=w537, y=3.141592653589793) -> (x/y=w539:dbl)
            n569 = Divide(x=w548, y=3.141592653589793) -> (x/y=w550:dbl)
            n570 = Power Of X(1:w539, 2:w540) -> (0:w542:dbl)
            n571 = Power Of X(1:w550, 2:w551) -> (0:w553:dbl)
            n572 = Multiply(x=w542, y=1000000.0) -> (x*y=w560:dbl)
            n573 = Multiply(x=w553, y=1000000.0) -> (x*y=w561:dbl)
            n574 = property on="Constrained Distribution" class="XYGraph (strict)"(error in=w557, "ActYScl"=1 ("Active Y Scale")) -> (error out=w559:errorcluster)  [unwired: 1 in, 1 out]
            n575 = property on="Constrained Distribution" class="XYGraph (strict)"(error in=w559, "YScale.Maximum"=w560, "YScale.Minimum"=w561) -> (error out=w565:errorcluster)  [unwired: 1 in, 1 out]
            n576 = property on="Constrained Distribution" class="XYGraph (strict)"(error in=w565, "YScale.MarkerVals[]"=dbl[] [0.01, 0.02, 0.05, 0.1, 0.2, 0.5, 1.0, 2.0, 5.0, 10.0] ("Y Scale.Marker Values[]")) -> (error out=w566:errorcluster)  [unwired: 1 in, 1 out]
            n577 = property on="Constrained Distribution" class="XYGraph (strict)"(error in=w566, "YScale.Visible"=TRUE ("Y Scale.Visible")) -> (error out=w563:errorcluster)  [unwired: 1 in, 1 out]
            n578 = property on="Constrained Distribution" class="XYGraph (strict)"(error in=w563, "ActYScl"=0 ("Active Y Scale")) -> (error out=w530:errorcluster)  [unwired: 1 in, 1 out]
            n579 = call <vilib>:"Clear Errors.vi"("error in (no error)"=w530) -> ()  [unwired: 6 in, 1 out]
          }
          frame True {
            n580 = property on="Constrained Distribution" class="XYGraph (strict)"("ActYScl"=1 ("Active Y Scale")) -> (error out=w582:errorcluster)  [unwired: 2 in, 1 out]
            n581 = property on="Radius (µm)" class="DigNum (strict)"("DisabledEnum"=T6."Disabled and Grayed Out" ("Disabled")) -> ()  [unwired: 2 in, 2 out]
            n582 = property on="Constrained Distribution" class="XYGraph (strict)"(error in=w582, "YScale.Visible"=FALSE ("Y Scale.Visible")) -> (error out=w583:errorcluster)  [unwired: 1 in, 1 out]
            n583 = property on="Constrained Distribution" class="XYGraph (strict)"(error in=w583, "ActYScl"=0 ("Active Y Scale")) -> ()  [unwired: 1 in, 2 out]
          }
        }
        n584 = case shown="True" "Reset Limit" {
          frame False {
          }
          frame True {
            n585 = local write "Throttle Dust Source After:"(inf) -> ()
          }
        }
        n586 = case shown="True" "Reset Scale to Default" {
          frame False {
          }
          frame True {
            n587 = property on="Constrained Distribution" class="XYGraph (strict)"("XScale.Maximum"=100.0 ("X Scale.Range:Maximum"), "XScale.Minimum"=0.1 ("X Scale.Range:Minimum"), "YScale.Maximum"=1e-10 ("Y Scale.Range:Maximum"), "YScale.Minimum"=1e-20 ("Y Scale.Range:Minimum")) -> ()  [unwired: 2 in, 2 out]
          }
        }
        n588 = property on="Save Waveforms" class="Bool (strict)"(error in=w516, "BoolText.Text"="Save Waveforms" ("f")) -> (error out=w514:errorcluster)  [unwired: 1 in, 1 out]
        n589 = property on="Save Metadata" class="Bool (strict)"(error in=w514, "BoolText.Text"="Save Metadata" ("Boolean Text.Text")) -> (error out=w513:errorcluster)  [unwired: 1 in, 1 out]
      }
      n590 = while {
        tunnel: [w159] -> w147
        tunnel: w145 -> [w158]
        tunnel: w146 -> [w155]
        stop <- w157 stop-if-true
        # "Real time plot update loop"
        n591 = local read "Update interval (s)"() -> (w156:dbl)
        n592 = Multiply(x=1000, y=w156) -> (x*y=w161:dbl)
        n593 = event shown="[0] Timeout;  \"Update Plot in Real-time?\": Value Change" {
          selector: _ -> [_ _ _ _ _]
          dyn-events: _ -> [_ _ _ _ _]
          timeout: w161 -> [_ _ _ _ _]
          tunnel: w158 -> [w178 w462 w467 w469 w494]
          tunnel: [w175 w461 w467 w476 w494] -> w160
          tunnel: [_ _ _ _ w493] -> w157
          tunnel: w155 -> [_ _ _ w490 _]
          event Timeout; "Update Plot in Real-time?": Value Change {
            n594 = event-data() -> ()  [unwired: 1 in, 2 out]
            n595 = property on="Plotted Experiment Groups" class="LstBox (strict)"() -> ("Item Names"=w169:string[])  [unwired: 2 in, 2 out]
            n596 = property on="Plotted Experiment Names" class="LstBox (strict)"() -> ("Item Names"=w174:string[])  [unwired: 2 in, 2 out]
            n597 = Array Size(array=w174) -> (size(s)=w173:i32)
            n598 = Array Size(array=w169) -> (size(s)=w171:i32)
            n599 = Less?(x=w173, y=3) -> (x < y?=w167:bool)
            n600 = Less?(x=w171, y=3) -> (x < y?=w168:bool)
            n601 = case shown="True" w167 {
              frame False {
              }
              frame True {
                n602 = property on="Plotted Experiment Names" class="LstBox (strict)"("Top Row"=0 ("Active Row:Active Row Number")) -> ()  [unwired: 2 in, 2 out]
              }
            }
            n603 = case shown="True" w168 {
              frame False {
              }
              frame True {
                n604 = property on="Plotted Experiment Groups" class="LstBox (strict)"("Top Row"=0 ("Active Row:Active Row Number")) -> ()  [unwired: 2 in, 2 out]
              }
            }
            n605 = call <userlib>:"Boolean Trigger__ogtk.vi"("Boolean Input"="Update Plot in Real-time?") -> ("Rising Edge"=w164:bool)  [unwired: 1 in, 1 out]
            n606 = First Call?() -> (First Call?: T/F=w165:bool)
            n607 = Or(x=w165, y=w164) -> (x .or. y?=w166:bool)
            n608 = Get Date/Time In Seconds() -> (seconds since 1Jan1904=w177:timestamp)
            n609 = case shown="True" "Update Plot in Real-time?" {
              tunnel: [w182 w289] -> w175
              tunnel: w178 -> [w188 w288]
              tunnel: w177 -> [_ w212]
              tunnel: T2 {"Upper Timestamp Range"=timestamp(0 s since 1904-01-01), "Lower Timestamp Range"=timestamp(0 s since 1904-01-01), "Experiment Group:"="", "Experiment Name:"=[], "Upper Velocity Limit (km/s)"=0.0, "Lower Velocity Limit (km/s)"=0.0, "Upper Mass Limit (kg)"=0.0, "Lower Mass Limit (kg)"=0.0, "name array"=[], "Estimate Quality"={0.0, 0.0}} ("Constraints 2") -> [_ w290]
              tunnel: w166 -> [_ w218]
              frame False {
                w181 = FALSE ("Visible")
                n610 = property on="Current Limits" class="Clust (strict)"("Visible"=FALSE) -> ()  [unwired: 2 in, 2 out]
                n611 = property on="Plot" class="Bool (strict)"("BoolText.Text"="Plot" ("Boolean Text.Text")) -> ()  [unwired: 2 in, 2 out]
                n612 = global write "throttle from query.vi" "Throttle Q"(FALSE ("Throttle Q")) -> ()
                n613 = property on="Throttle Dust Source After:" class="DigNum (strict)"(error in=w188, "Visible"=w181) -> (error out=w183:errorcluster)  [unwired: 1 in, 1 out]
                n614 = local write "Throttle Dust Source After:"(inf) -> ()
                n615 = property on="Reset Limit" class="Bool"(error in=w183, "Visible"=w181) -> (error out=w182:errorcluster)  [unwired: 1 in, 1 out]
              }
              frame True {
                w258 = 0 ("index (row)")
                w252 = ""
                w197 = TRUE ("Visible")
                n616 = local read "Plotted Cluster"() -> (w225:T2)
                n617 = property on="Upper Timestamp Range" class="AbsTime (strict)"(error in=w288, "Value"=w212) -> (error out=w283:errorcluster)  [unwired: 1 in, 1 out]
                n618 = Select(t=T2 {"Upper Timestamp Range"=timestamp(0 s since 1904-01-01), "Lower Timestamp Range"=timestamp(0 s since 1904-01-01), "Experiment Group:"="", "Experiment Name:"=[], "Upper Velocity Limit (km/s)"=299800.0, "Lower Velocity Limit (km/s)"=0.0, "Upper Mass Limit (kg)"=1.0, "Lower Mass Limit (kg)"=0.0, "name array"=[], "Estimate Quality"={2.0, 5.0}}, s=w218, f=w225) -> (s? t:f=w224:T2)
                n619 = Unbundle By Name(w224) -> ("Lower Timestamp Range"=w211:timestamp, "Experiment Name:"=w253:i32[], "Upper Velocity Limit (km/s)"=w210:dbl, "Lower Velocity Limit (km/s)"=w209:dbl, "Upper Mass Limit (kg)"=w208:dbl, "Lower Mass Limit (kg)"=w207:dbl, "Estimate Quality"=w195:cluster{dbl, dbl})
                n620 = Bundle("Lower Timestamp Range"=w211, "Upper Velocity Limit (km/s)"=w210, "Lower Velocity Limit (km/s)"=w209, "Upper Mass Limit (kg)"=w208, "Lower Mass Limit (kg)"=w207, "Estimate Quality"=w195) -> (→"Current Limits":T19)  [unwired: 1 in]
                n621 = call "connect in.vi"() -> ("error out"=w204:errorcluster, "Database Connection"=w266:T12)  [unwired: 7 in, 1 out]
                n622 = call-poly <vilib>:"DB Tools Execute Query.vi"("error in (no error)"=w204, "cursor type"=DB_Tools_Cursor_Type."dynamic", "SQL query"="SELECT tag,groups.group_names FROM `CCLDAS_PRODUCTION`.`experiment_settings`\nINNER JOIN\ngroups ON experiment_settings.id_groups = groups.id_groups\n\nORDER BY id_experiment_settings DESC LIMIT 1;", "connection reference"=w266) -> ("error out"=w263:errorcluster, "recordset reference"=w262:T13)  [unwired: 4 in]
                n623 = call-poly <vilib>:"DB Tools Fetch Recordset Data.vi"("error in (no error)"=w263, "recordset reference"=w262) -> ("error out"=w254:errorcluster, "recordset data"=w260:variant[][], "recordset reference out"=w261:T13)  [unwired: 3 in]
                n624 = call-poly <vilib>:"DB Tools Free Object.vi"("error in (no error)"=w254, "recordset reference"=w261) -> ("error out"=w201:errorcluster, "connection reference"=w251:T12)  [unwired: 8 in]
                n625 = Index Array(array=w260, index (row) #1=w258, index (col) #1=0 ("disabled index (col)"), index (row) #2=w258, index (col) #2=1 ("disabled index (col)")) -> (element #1=w256:variant, element #2=w255:variant)
                n626 = call "connect out.vi"("error in (no error)"=w204, "connection reference"=w251) -> ("error out"=w250:errorcluster)  [unwired: 9 in]
                n627 = property on="Current Limits" class="Clust (strict)"("Visible"=TRUE) -> ()  [unwired: 2 in, 2 out]
                n628 = property on="Plot" class="Bool (strict)"("BoolText.Text"="Limit" ("Boolean Text.Text")) -> ()  [unwired: 2 in, 2 out]
                n629 = xnode "Database Variant To Data"("database variant"=w255, "error in (no error)"=w250, "type"=w252) -> ("data"=w223:string, "error out"=w202:errorcluster)
                n630 = xnode "Database Variant To Data"("database variant"=w256, "error in (no error)"=w250, "type"=w252) -> ("data"=w235:string, "error out"=w203:errorcluster)
                n631 = Build Array(w235) -> (w194:string[])
                n632 = call-poly <userlib>:"Data Changed__ogtk.vi"("1D String Array"=w194) -> ("Changed"=w198:bool)
                n633 = Or(x=w198, y=w218) -> (x .or. y?=w199:bool)
                n634 = Bundle By Name(cluster=w290, "Upper Timestamp Range"=w212, "Lower Timestamp Range"=w211, "Experiment Group:"=w223, "Experiment Name:"=w253, "Upper Velocity Limit (km/s)"=w210, "Lower Velocity Limit (km/s)"=w209, "Upper Mass Limit (kg)"=w208, "Lower Mass Limit (kg)"=w207, "name array"=w194, "Estimate Quality"=w195) -> (w193:T2)
                "Plotted Cluster" <- w193
                n635 = case shown="True" w199 {
                  tunnel: w194 -> [_ w296]
                  tunnel: w223 -> [_ w297]
                  tunnel: [errorcluster {"status"=FALSE, "code"=0, "source"=""} ("error out") w294] -> w214
                  tunnel: [errorcluster {"status"=FALSE, "code"=0, "source"=""} ("error out") w293] -> w213
                  frame False {
                  }
                  frame True {
                    n636 = Build Array(w297) -> (w295:string[])
                    n637 = property on="Groups to add" class="Arr (strict)"("Value"=w295) -> (error out=w293:errorcluster)  [unwired: 2 in, 1 out]
                    n638 = property on="Experiments to add" class="Arr (strict)"("Value"=w296) -> (error out=w294:errorcluster)  [unwired: 2 in, 1 out]
                  }
                }
                n639 = Merge Errors(w203, w202, w201) -> (w200:errorcluster)
                n640 = call <vilib>:"Clear Errors.vi"("error in (no error)"=w200) -> ()  [unwired: 6 in, 1 out]
                n641 = call "Get_Groups_And_Names.vi"("error in (no error)"=w283, "Constraints"=w193) -> ("error out"=w274:errorcluster, "Description"=w277:string[], "Groups"=w282:string[], "Description Returned?"=w281:bool, "Run start integer timestamp"=w276:i64[], "Run Time (hrs)"=w196:string[], "Run stop integer timesamp"=w275:i64[])  [unwired: 2 in, 1 out]
                n642 = for {
                  tunnel: w277 -> [w435] mode=indexing
                  tunnel: w276 -> [w450] mode=indexing
                  tunnel: w275 -> [w451] mode=indexing
                  shift-right: [w437] -> w273
                  shift-left: w274 -> [w448]
                  shift-right: [w439] -> w238
                  shift-left: _ -> [w436]
                  tunnel: w196 -> [w433] mode=indexing
                  i -> [w442]
                  n643 = Concatenate Strings(w436, w435) -> (w434:string)
                  n644 = call "timestamp_reversion.vi"("error in (no error)"=w448, "Integer Timestamp"=w450) -> ("error out"=w449:errorcluster, "time stamp"=w446:timestamp)  [unwired: 7 in]
                  n645 = call "timestamp_reversion.vi"("error in (no error)"=w449, "Integer Timestamp"=w451) -> ("error out"=w438:errorcluster, "time stamp"=w447:timestamp)  [unwired: 7 in]
                  n646 = Equal To 0?(x=w442) -> (x = 0?=w440:bool)
                  n647 = Format Date/Time String(seconds (now)=w447) -> (date/time string=w443:string)  [unwired: 2 in]
                  n648 = Select(t=w435, s=w440, f=w434) -> (s? t:f=w441:string)
                  n649 = Format Date/Time String(seconds (now)=w446) -> (date/time string=w444:string)  [unwired: 2 in]
                  n650 = Format Into String(format string="%s\nRun from %s to %s for %s hours.\n", error in=w438, w441, w444, w443, w433) -> (resulting string=w439:string, error out=w437:errorcluster)  [unwired: 1 in]
                }
                n651 = property on="Description for Experiment Name:" class="Str"(error in=w273, "Visible"=w281) -> (error out=w280:errorcluster)  [unwired: 1 in, 1 out]
                n652 = property on="Experiment Group:" class="CmbBox"(error in=w280, "Strings[]"=w282) -> (error out=w269:errorcluster)  [unwired: 1 in, 1 out]
                n653 = property on="Description for Experiment Name:" class="Str"(error in=w269, "Caption.Text"="Experiment Description:" ("format string")) -> (error out=w279:errorcluster)  [unwired: 1 in, 1 out]
                n654 = property on="Throttle Dust Source After:" class="DigNum (strict)"("Visible"=w197) -> ()  [unwired: 2 in, 2 out]
                n655 = property on="Groups to add" class="Arr (strict)"(error in=w213) -> ("Value"=w215:string[])  [unwired: 1 in, 2 out]
                n656 = property on="Experiments\nto add" class="Arr (strict)"(error in=w214) -> ("Value"=w216:string[])  [unwired: 1 in, 2 out]
                n657 = property on="Reset Limit" class="Bool"("Visible"=w197) -> ()  [unwired: 2 in, 2 out]
                n658 = Delete From Array(array=w215, index=0) -> (array with subset deleted=w220:string[])  [unwired: 1 in, 1 out]
                n659 = Format Into String(format string="Experiment Group: %s\n%s", w223, w238) -> (resulting string=w237:string)  [unwired: 2 in, 1 out]
                n660 = Build Array (concatenate)(w223, w220) -> (w241:string[])
                n661 = Delete From Array(array=w216, index=0) -> (array with subset deleted=w222:string[])  [unwired: 1 in, 1 out]
                n662 = call "read_db_for_plot.vi"("error in (no error)"=w279, "Constraints 2"=w193) -> ("error out"=w245:errorcluster, "Total Number of events"=w217:i64, "Dust Array"=w247:T7[], "Dust Info"=w234:cluster{"Density":dbl, "Name":string}[])  [unwired: 5 in, 1 out]
                n663 = call-poly <userlib>:"Remove Duplicates from 1D Array__ogtk.vi"("Input Array"=w241) -> ("Output Array"=w240:string[])  [unwired: 1 out]
                n664 = property on="Plotted Experiment Groups" class="LstBox (strict)"("Item Names"=w240) -> ()  [unwired: 2 in, 2 out]
                n665 = call-poly <userlib>:"Remove Duplicates from 1D Array__ogtk.vi"("Input Array"=w220) -> ("Output Array"=w248:string[])  [unwired: 1 out]
                n666 = Build Array (concatenate)(w235, w222) -> (w236:string[])
                n667 = property on="Plotted Experiment Names" class="LstBox (strict)"("Item Names"=w236) -> ()  [unwired: 2 in, 2 out]
                n668 = Index Array(array=w234) -> (element=w233:cluster{"Density":dbl, "Name":string})  [unwired: 1 in]
                n669 = Unbundle By Name(w233) -> ("Density"=w227:dbl, "Name"=w230:string)
                n670 = for {
                  tunnel: w248 -> [w322] mode=indexing
                  tunnel: w220 -> [w305]
                  tunnel: w222 -> [w304]
                  shift-right: [w340] -> w246
                  shift-left: w247 -> [w341]
                  tunnel: [w321] -> w242 mode=indexing
                  tunnel: w193 -> [w302]
                  tunnel: w230 -> [w315]
                  shift-right: [w314] -> w231
                  shift-left: TRUE -> [w320]
                  shift-right: [w313] -> w191
                  shift-left: w217 -> [w301]
                  shift-right: [w328] -> w244
                  shift-left: w245 -> [w303]
                  w306 = "Any Experiment."
                  n671 = call-poly <userlib>:"Search Array__ogtk.vi"("Array"=w305, "Element Data"=w322) -> ("Indices of Elements"=w342:i32[])  [unwired: 7 in]
                  n672 = call-poly <userlib>:"Index Array Elements__ogtk.vi"("indices"=w342, "array"=w304) -> ("elements"=w310:string[])  [unwired: 9 in]
                  n673 = Equal?(x=w310, y=w306) -> (x = y?=w312:bool[])
                  n674 = Or Array Elements(Boolean array=w312) -> (logical OR=w311:bool)
                  n675 = Build Array(w306) -> (w309:string[])
                  n676 = Unbundle(w302) -> ("Upper Timestamp Range"=w339:timestamp, "Lower Timestamp Range"=w338:timestamp, "Experiment Name:"=w337:i32[], "Upper Velocity Limit (km/s)"=w336:dbl, "Lower Velocity Limit (km/s)"=w335:dbl, "Upper Mass Limit (kg)"=w334:dbl, "Lower Mass Limit (kg)"=w333:dbl, "name array"=w332:string[], "Estimate Quality"=w298:cluster{dbl, dbl})  [unwired: 1 out]
                  n677 = Select(t=w309, s=w311, f=w310) -> ()  [unwired: 1 out]
                  n678 = Bundle(cluster=w302, "Upper Timestamp Range"=w339, "Lower Timestamp Range"=w338, "Experiment Group:"=w322, "Experiment Name:"=w337, "Upper Velocity Limit (km/s)"=w336, "Lower Velocity Limit (km/s)"=w335, "Upper Mass Limit (kg)"=w334, "Lower Mass Limit (kg)"=w333, "name array"=w332, "Estimate Quality"=w298) -> (w331:T2)
                  n679 = call "read_db_for_plot.vi"("error in (no error)"=w303, "Constraints 2"=w331) -> ("error out"=w330:errorcluster, "Total Number of events"=w300:i64, "Dust Array"=w299:T7[], "Dust Info"=w316:cluster{"Density":dbl, "Name":string}[])  [unwired: 5 in, 1 out]
                  n680 = call "Get_Groups_And_Names.vi"("error in (no error)"=w330, "Constraints"=w331) -> ("error out"=w329:errorcluster, "Description"=w325:string[], "Run start integer timestamp"=w327:i64[], "Run Time (hrs)"=w307:string[], "Run stop integer timesamp"=w326:i64[])  [unwired: 2 in, 3 out]
                  n681 = for {
                    tunnel: w325 -> [w352] mode=indexing
                    tunnel: w327 -> [w367] mode=indexing
                    tunnel: w326 -> [w368] mode=indexing
                    shift-right: [w354] -> w328
                    shift-left: w329 -> [w365]
                    shift-right: [w356] -> w324
                    shift-left: _ -> [w353]
                    tunnel: w307 -> [w350] mode=indexing
                    i -> [w359]
                    n682 = Concatenate Strings(w353, w352) -> (w351:string)
                    n683 = call "timestamp_reversion.vi"("error in (no error)"=w365, "Integer Timestamp"=w367) -> ("error out"=w366:errorcluster, "time stamp"=w363:timestamp)  [unwired: 7 in]
                    n684 = call "timestamp_reversion.vi"("error in (no error)"=w366, "Integer Timestamp"=w368) -> ("error out"=w355:errorcluster, "time stamp"=w364:timestamp)  [unwired: 7 in]
                    n685 = Equal To 0?(x=w359) -> (x = 0?=w357:bool)
                    n686 = Select(t=w352, s=w357, f=w351) -> (s? t:f=w358:string)
                    n687 = Format Date/Time String(seconds (now)=w363) -> (date/time string=w361:string)  [unwired: 2 in]
                    n688 = Format Date/Time String(seconds (now)=w364) -> (date/time string=w360:string)  [unwired: 2 in]
                    n689 = Format Into String(format string="%s\nRun from %s to %s for %s hrs.\n", error in=w355, w358, w361, w360, w350) -> (resulting string=w356:string, error out=w354:errorcluster)  [unwired: 1 in]
                  }
                  n690 = Build Array (concatenate)(w341, w299) -> (w340:T7[])
                  n691 = Array Size(array=w316) -> (size(s)=w308:i32)
                  n692 = Add(x=w300, y=w301) -> (x+y=w313:i64)
                  n693 = Equal?(x=w308, y=1) -> (x = y?=w319:bool)
                  n694 = And(x=w320, y=w319) -> (x .and. y?=w317:bool)
                  n695 = case shown="True" w317 {
                    tunnel: w316 -> [_ w349]
                    tunnel: w315 -> [_ w346]
                    tunnel: [w343 w345] -> w314
                    tunnel: w308 -> [w344 _]
                    frame False {
                      n696 = Equal To 0?(x=w344) -> (x = 0?=w343:bool)
                    }
                    frame True {
                      n697 = Index Array(array=w349) -> (element=w348:cluster{"Density":dbl, "Name":string})  [unwired: 1 in]
                      n698 = Unbundle By Name(w348) -> ("Name"=w347:string)
                      n699 = Equal?(x=w346, y=w347) -> (x = y?=w345:bool)
                    }
                  }
                  n700 = Format Into String(format string="\nExperiment Group: %s\n%s", w322, w324) -> (resulting string=w321:string)  [unwired: 2 in, 1 out]
                }
                n701 = Multiply(x=1000.0, y=w227) -> (x*y=w190:dbl)
                n702 = local write "Density"(w190) -> ()
                n703 = Select(t=w230, s=w231, f="Multiple Dust Type" ("t")) -> (s? t:f=w228:string)
                n704 = local write "Dust Type"(w228) -> ()
                n705 = Concatenate Strings(w237, w242) -> (w243:string)
                n706 = local write "Description for Experiment Name:"(w243) -> ()
                n707 = local read "Vnoise Estimate:"() -> (w285:dbl)
                n708 = local write "Total Number of triggers:"(w191) -> ()
                n709 = local read "Sensitivity:"() -> (w286:dbl)
                n710 = local read "Pelletron Voltage (MV):"() -> (w284:dbl)
                n711 = call "generate_plot.vi"("High Voltage"=w284, "Sens"=w286, "error in"=w244, "Vnoise"=w285, "Dust Array"=w246) -> ("error out"=w289:errorcluster, "Number of matching good events"=w192:i32, "Dust Distribution"=w287:T4)  [unwired: 4 in]
                n712 = local write "Number of Matching Events:"(w192) -> ()
                n713 = Divide(x=w192, y=w191) -> (x/y=w271:dbl)
                n714 = Multiply(x=w271, y=100.0) -> (x*y=w270:dbl)
                n715 = local write "Percentage of triggers that fit constraints:"(w270) -> ()
                n716 = local write "Constrained Distribution"(w287) -> ()
                n717 = Greater Or Equal?(x=w192, y="Throttle Dust Source After:") -> (x >= y?=w268:bool)
                n718 = global write "throttle from query.vi" "Throttle Q"(w268) -> ()
              }
            }
          }
          event "Clear Extra Plots": Value Change {
            n719 = event-data() -> ()  [unwired: 1 in, 5 out]
            n720 = local read "Update Plot in Real-time?"() -> (w460:bool)
            n721 = case shown="True" w460 {
              tunnel: w462 -> [w463 w466]
              tunnel: [w463 w465] -> w461
              frame False {
              }
              frame True {
                n722 = property on="Update Plot in Real-time?" class="Bool (strict)"(error in=w466, "Val(Sgnl)"=TRUE ("Value (Signaling)")) -> (error out=w465:errorcluster)  [unwired: 1 in, 1 out]
              }
            }
            n723 = local read "Experiments\nto add"() -> (w457:string[])
            n724 = local read "Groups to add"() -> (w459:string[])
            n725 = Index Array(array=w459, index=0) -> (element=w454:string)
            n726 = Index Array(array=w457, index=0) -> (element=w455:string)
            n727 = Build Array(w454) -> (w453:string[])
            n728 = Build Array(w455) -> (w452:string[])
            n729 = local write "Experiments\nto add"(w452) -> ()
            n730 = local write "Groups to add"(w453) -> ()
          }
          event "Update interval (s)": Value Change {
            n731 = event-data() -> ()  [unwired: 1 in, 5 out]
          }
          event "Reset Constraints to Default": Value Change {
            w470 = FALSE ("Visible")
            w474 = ""
            n732 = event-data() -> ()  [unwired: 1 in, 5 out]
            n733 = Unbundle By Name(w490) -> ("Experiment Group:"=w489:string, "Experiment Name:"=w488:i32[], "Upper Velocity Limit (km/s)"=w487:dbl, "Lower Velocity Limit (km/s)"=w486:dbl, "Upper Mass Limit (kg)"=w485:dbl, "Lower Mass Limit (kg)"=w484:dbl, "name array"=w478:string[], "Estimate Quality"=w468:cluster{dbl, dbl})  [unwired: 1 out]
            n734 = Get Date/Time In Seconds() -> (seconds since 1Jan1904=w483:timestamp)
            n735 = Bundle By Name(cluster=w490, "Upper Timestamp Range"=w483, "Lower Timestamp Range"=timestamp(0 s since 1904-01-01), "Experiment Group:"=w489, "Experiment Name:"=w488, "Upper Velocity Limit (km/s)"=w487, "Lower Velocity Limit (km/s)"=w486, "Upper Mass Limit (kg)"=w485, "Lower Mass Limit (kg)"=w484, "name array"=w478, "Estimate Quality"=w468) -> (w482:T2)
            n736 = property on="Experiment Name:" class="LstBox (strict)"("ColHdr"="Any Experiment." ("element")) -> ()  [unwired: 2 in, 2 out]
            n737 = local write "Constraints"(w482) -> ()
            n738 = local write "Experiment Name"(w474) -> ()
            n739 = local write "Experiment Group"(w474) -> ()
            n740 = flat-sequence {
              frame #0 {
                n741 = Wait (ms)(milliseconds to wait=u32 100) -> ()  [unwired: 1 out]
              }
              frame #1 {
                n742 = local write "Reset Constraints to Default"(FALSE ("Reset Constraints to Default")) -> ()
              }
            }
            n743 = property on="Show Names" class="Bool (strict)"("Visible"=TRUE, "Value"=w470) -> ()  [unwired: 2 in, 2 out]
            n744 = call "Get_Groups_And_Names.vi"("error in (no error)"=w469, "Constraints"=w482) -> ("error out"=w479:errorcluster, "Groups"=w481:string[], "Names"=w480:string[])  [unwired: 2 in, 5 out]
            n745 = local write "Names"(w480) -> ()
            n746 = property on="Experiment Group:" class="CmbBox"(error in=w479, "Strings[]"=w481) -> (error out=w476:errorcluster)  [unwired: 1 in, 1 out]
            n747 = property on="Select Names" class="Bool (strict)"("Visible"=w470, "Value"=w470) -> ()  [unwired: 2 in, 2 out]
            n748 = property on="Experiment Name:" class="LstBox (strict)"("Height"=u32 25 ("Size:Height")) -> ()  [unwired: 2 in, 2 out]
            "Reset" <- FALSE
          }
          event "Exit": Value Change {
            n749 = event-data() -> ()  [unwired: 1 in, 5 out]
            n750 = local read "Exit"() -> (w493:bool)
          }
        }
        n751 = Merge Errors(w158, w160) -> (w159:errorcluster)
      }
      n752 = for {
        tunnel: w144 -> [w154] mode=indexing
        tunnel: w143 -> [w153]
        tunnel: [w152] -> w142
        n753 = invoke class="VI" method="FP.Close"(reference=w154, error in=w153) -> (error out=w152:errorcluster)  [unwired: 1 in, 2 out]
      }
      n754 = Merge Errors(w143, w147, w142) -> (w148:errorcluster)
    }
    frame Error {
    }
  }
  "error out" <- w89
  n755 = Multiply(x=w49, y=100.0) -> (x*y=w50:dbl)
  n756 = local write "Percentage of triggers that fit constraints:"(w50) -> ()
